vi "Checkers PvP With File Loading.vi"() -> ()   [LabVIEW 2016]
uses:
  <vilib>/Utility/miscctls.llb/LVPositionTypeDef.ctl
  Game Info Global Variable.vi
  Board Layout Global Variable.vi
panel:
  out "P2 Bottom Right Marker":picture
  out "P2 Bottom Left Marker":picture
  out "P2 Top Left Marker":picture
  out "P2 Top Right Marker":picture
  out "P1 Bottom Left Marker":picture
  out "P1 Bottom Right Marker":picture
  out "P1 Top Right Marker":picture
  out "P1 Top Left Marker":picture
  in  "Save and Quit":bool
  out "Player 2 Name":string="Player 2"
  out "Player 1 Name":string="Player 1"
  out "P2 King 12":picture
  out "P2 King 11":picture
  out "P2 King 10":picture
  out "P2 King 9":picture
  out "P2 King 8":picture
  out "P2 King 7":picture
  out "P2 King 6":picture
  out "P2 King 5":picture
  out "P2 King 4":picture
  out "P2 King 3":picture
  out "P2 King 2":picture
  out "P2 King":picture
  out "P1 King 12":picture
  out "P1 King 11":picture
  out "P1 King 10":picture
  out "P1 King 9":picture
  out "P1 King 8":picture
  out "P1 King 7":picture
  out "P1 King 6":picture
  out "P1 King 5":picture
  out "P1 King 4":picture
  out "P1 King 3":picture
  out "P1 King 2":picture
  out "P1 King":picture
  out "P2 Piece Icon":picture
  out "P1 Piece Icon":picture
  out "P2 Piece 12":picture
  out "P2 Piece 11":picture
  out "P2 Piece 10":picture
  out "P2 Piece 9":picture
  out "P2 Piece 8":picture
  out "P2 Piece 7":picture
  out "P2 Piece 6":picture
  out "P2 Piece 5":picture
  out "P2 Piece 4":picture
  out "P2 Piece 3":picture
  out "P2 Piece 2":picture
  out "P1 Piece 12":picture caption="P1 Piece"
  out "P1 Piece 11":picture caption="P1 Piece"
  out "P1 Piece 10":picture caption="P1 Piece"
  out "P1 Piece 9":picture caption="P1 Piece"
  out "P1 Piece 8":picture caption="P1 Piece"
  out "P1 Piece 7":picture caption="P1 Piece"
  out "P1 Piece 6":picture caption="P1 Piece"
  out "P1 Piece 5":picture caption="P1 Piece"
  out "P1 Piece 4":picture caption="P1 Piece"
  out "P1 Piece 3":picture caption="P1 Piece"
  out "P2 Piece":picture
  out "P1 Piece 2":picture caption="P1 Piece"
  out "Game String":string
  out "P2 Turn Light":bool
  out "P1 Turn Light":bool=TRUE
  out "P1 Piece":picture
  in  "Offer Draw":bool
  in  "Surrender":bool
  out "Player 2 Label":string="Player 1"
  out "Player 1 Label":string="Player 1"
  in  "Save":bool
  in  "Quit":bool
  # "Your Turn!"
  # "Your Turn!"
  # "678, \n308"
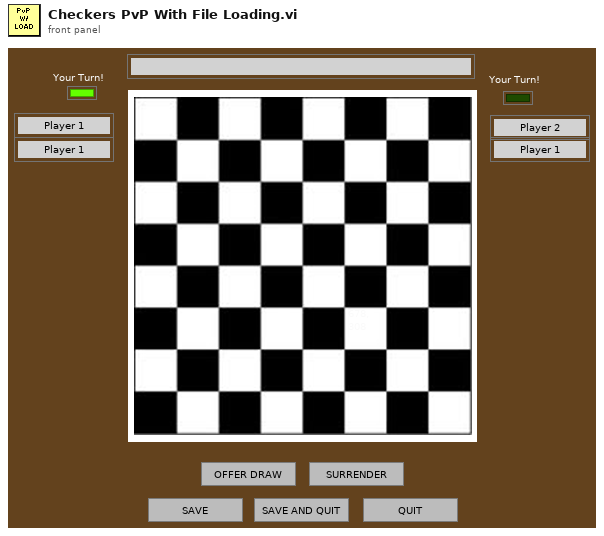
[diagram p1: front panel]
types:
  T1 = typedef "LVPositionTypeDef.ctl" = cluster{"Left":i32, "Top":i32}
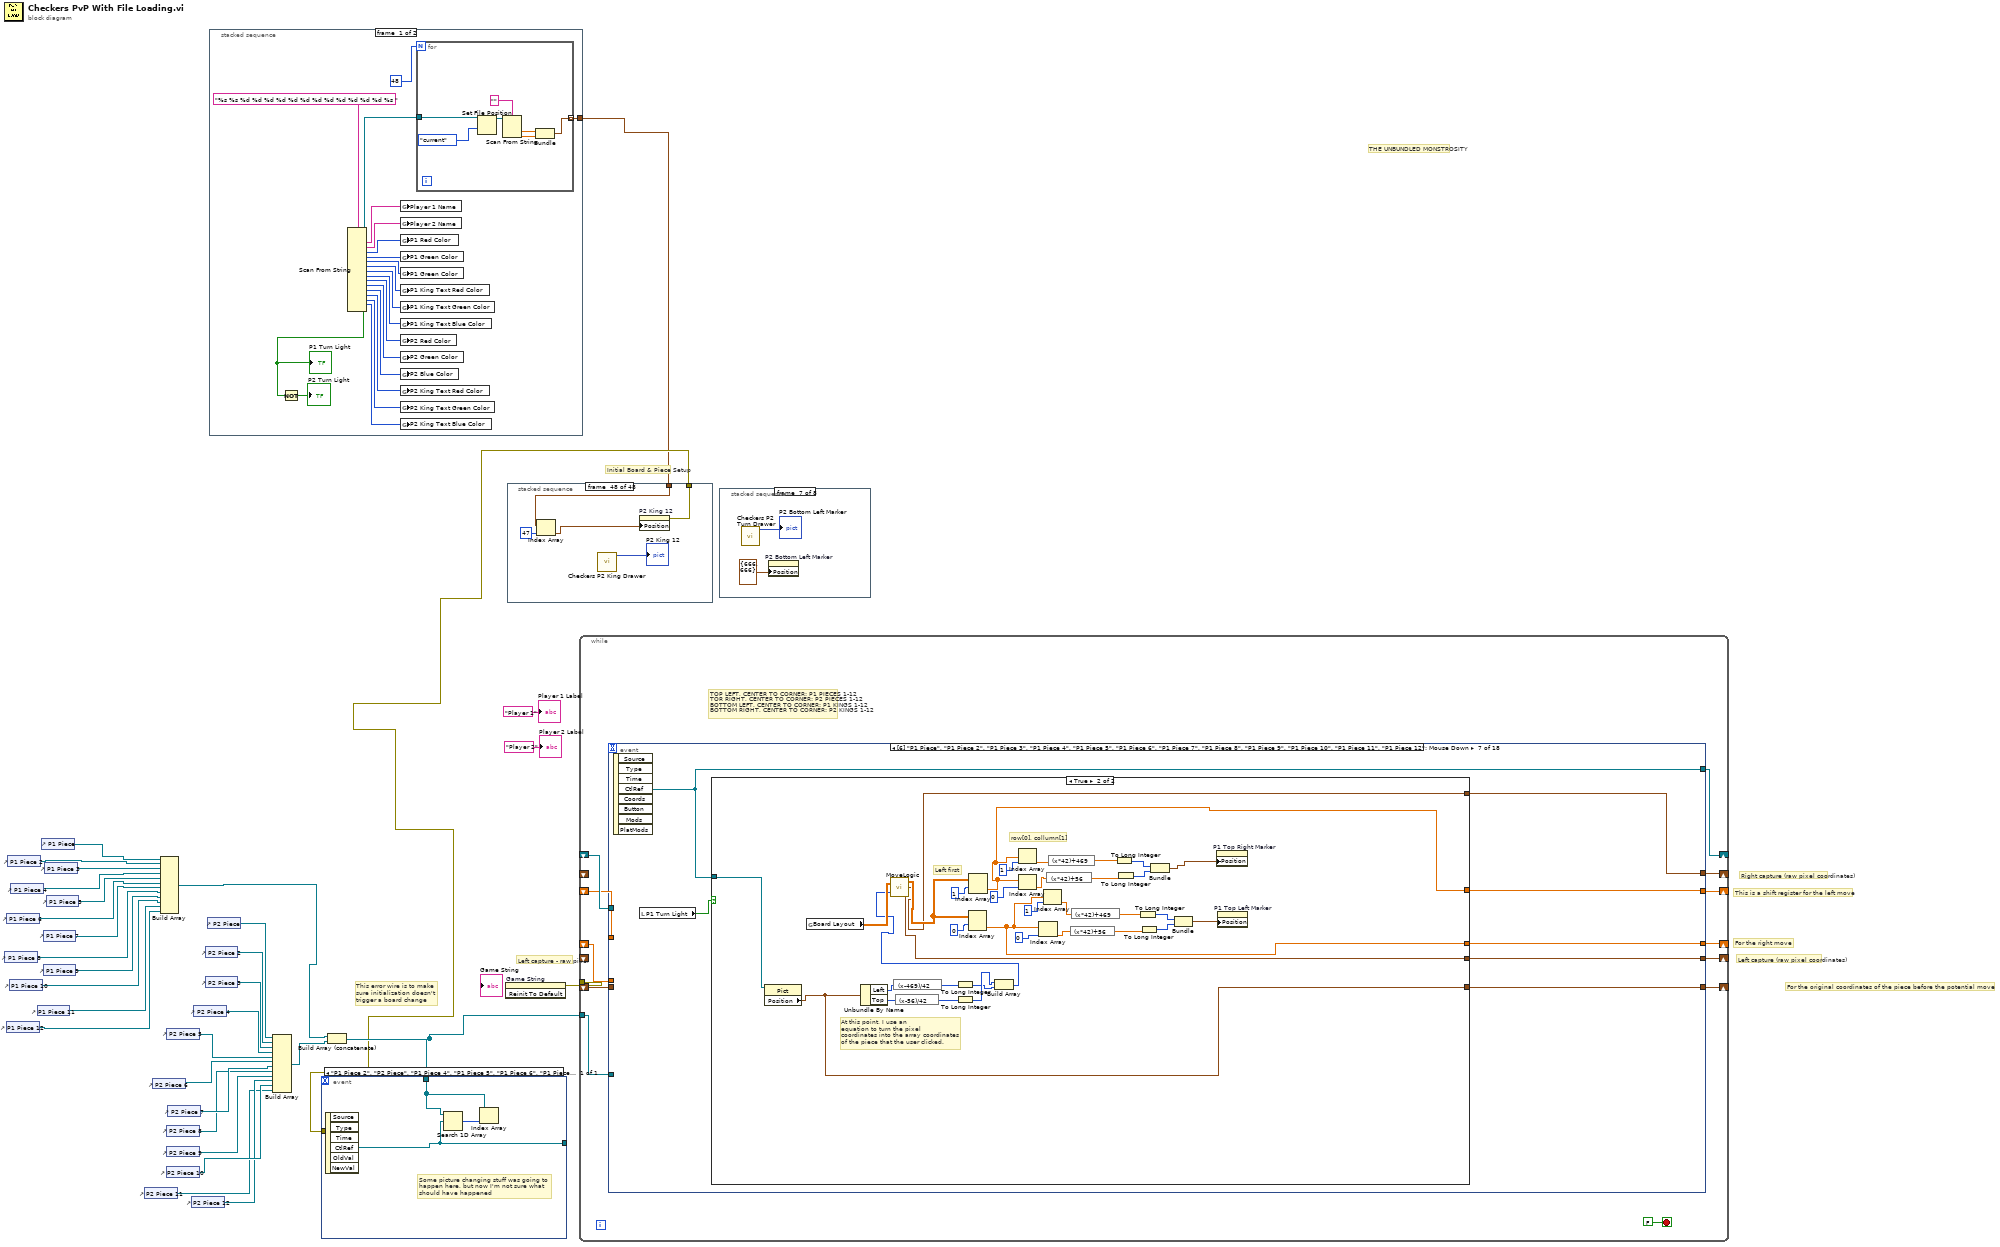
[diagram p0: block diagram]
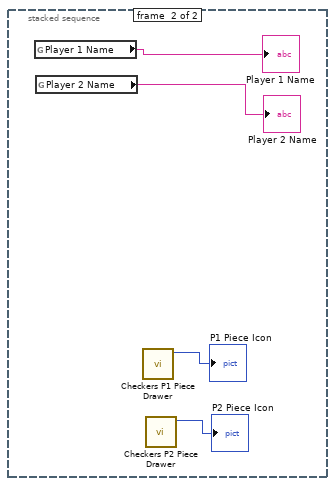
[diagram p2: hidden frame]
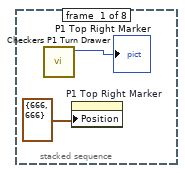
[diagram p3: hidden frame]
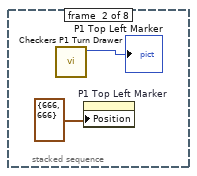
[diagram p4: hidden frame]
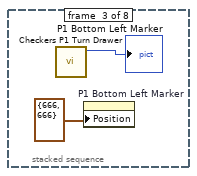
[diagram p5: hidden frame]
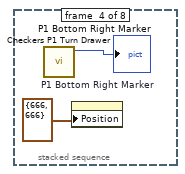
[diagram p6: hidden frame]
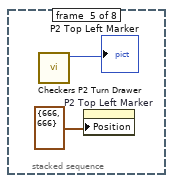
[diagram p7: hidden frame]
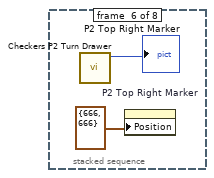
[diagram p8: hidden frame]
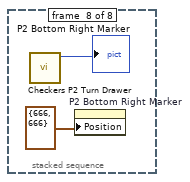
[diagram p9: hidden frame]
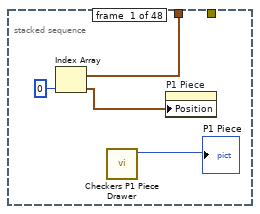
[diagram p10: hidden frame]
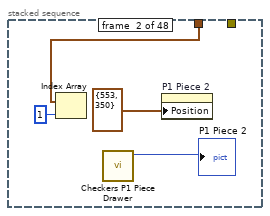
[diagram p11: hidden frame]
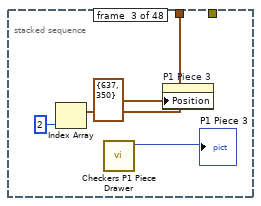
[diagram p12: hidden frame]
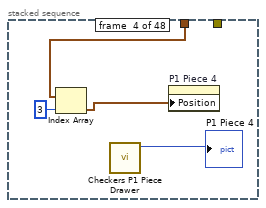
[diagram p13: hidden frame]
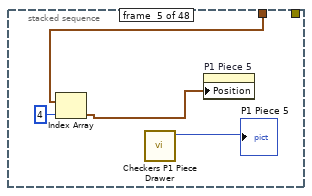
[diagram p14: hidden frame]
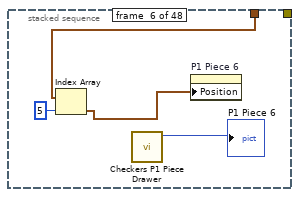
[diagram p15: hidden frame]
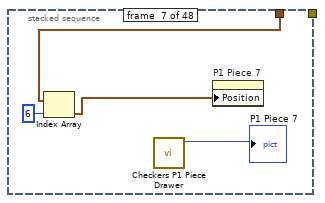
[diagram p16: hidden frame]
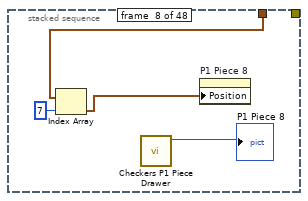
[diagram p17: hidden frame]
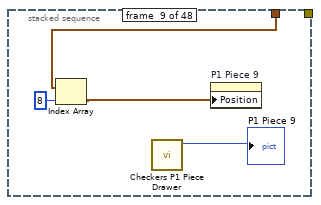
[diagram p18: hidden frame]
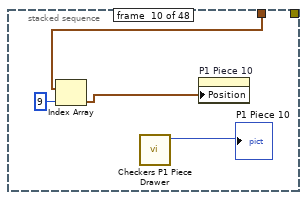
[diagram p19: hidden frame]
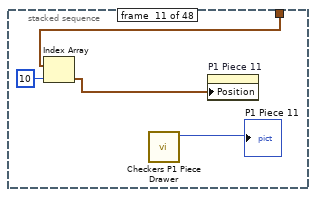
[diagram p20: hidden frame]
diagram:
  # "Left capture - raw pixel"
  # "Right capture (raw pixel coordinates)"
  # "Left capture (raw pixel coordinates)"
  # "For the original coordinates of the piece before the potential move"
  # "For the right move"
  # "This error wire is to make \nsure initialization doesn't \ntrigger a board change"
  # "This is a shift register for the left move"
  # "THE UNBUNDLED MONSTROSITY"
  # "Initial Board & Piece Setup"
  n1 = control-ref of="P1 Piece 8"() -> (w19:refnum<vi>)
  n2 = control-ref of="P1 Piece 6"() -> (w21:refnum<vi>)
  n3 = control-ref of="P1 Piece 12"() -> (w15:refnum<vi>)
  n4 = control-ref of="P1 Piece 2"() -> (w25:refnum<vi>)
  n5 = control-ref of="P1 Piece 10"() -> (w17:refnum<vi>)
  n6 = control-ref of="P1 Piece 4"() -> (w23:refnum<vi>)
  n7 = control-ref of="P1 Piece 11"() -> (w16:refnum<vi>)
  n8 = control-ref of="P1 Piece"() -> (w26:refnum<vi>)
  n9 = control-ref of="P1 Piece 7"() -> (w20:refnum<vi>)
  n10 = control-ref of="P1 Piece 9"() -> (w18:refnum<vi>)
  n11 = control-ref of="P1 Piece 3"() -> (w24:refnum<vi>)
  n12 = control-ref of="P1 Piece 5"() -> (w22:refnum<vi>)
  n13 = control-ref of="P2 Piece 11"() -> (w3:refnum<vi>)
  n14 = control-ref of="P2 Piece 6"() -> (w9:refnum<vi>)
  n15 = Build Array(w26, w25, w24, w23, w22, w21, w20, w19, w18, w17, w16, w15) -> (w2:refnum<vi>[])
  n16 = control-ref of="P2 Piece 5"() -> (w10:refnum<vi>)
  n17 = control-ref of="P2 Piece 8"() -> (w7:refnum<vi>)
  n18 = control-ref of="P2 Piece 9"() -> (w6:refnum<vi>)
  n19 = control-ref of="P2 Piece 10"() -> (w5:refnum<vi>)
  n20 = control-ref of="P2 Piece 7"() -> (w8:refnum<vi>)
  n21 = control-ref of="P2 Piece 12"() -> (w4:refnum<vi>)
  n22 = control-ref of="P2 Piece 4"() -> (w11:refnum<vi>)
  n23 = control-ref of="P2 Piece 2"() -> (w13:refnum<vi>)
  n24 = control-ref of="P2 Piece 3"() -> (w12:refnum<vi>)
  n25 = control-ref of="P2 Piece"() -> (w14:refnum<vi>)
  n26 = stacked-sequence {
    tunnel: [w35 _] -> w1
    frame #0 {
      n27 = Scan From String("%s %s %d %d %d %d %d %d %d %d %d %d %d %d %s " ("format string")) -> (w51:refnum<file>, output 1=w49:string, output 2=w48:string, output 3=w47:i32, output 4=w46:i32, output 5=w45:i32, output 6=w44:i32, output 7=w43:i32, output 8=w42:i32, output 9=w41:i32, output 10=w40:i32, output 11=w39:i32, output 12=w38:i32, output 13=w37:i32, output 14=w36:i32, output 15=w33:bool)  [unwired: 17 in, 1 out]
      "P1 Turn Light" <- w33
      n28 = Not(x=w33) -> (.not. x?=→"P2 Turn Light":bool)
      n29 = global write "Game Info Global Variable.vi" "Player 1 Name"(w49) -> ()
      n30 = global write "Game Info Global Variable.vi" "Player 2 Name"(w48) -> ()
      n31 = global write "Game Info Global Variable.vi" "P1 Red Color"(w47) -> ()
      n32 = global write "Game Info Global Variable.vi" "P1 Green Color"(w46) -> ()
      n33 = global write "Game Info Global Variable.vi" "P1 Green Color"(w45) -> ()
      n34 = global write "Game Info Global Variable.vi" "P1 King Text Red Color"(w44) -> ()
      n35 = global write "Game Info Global Variable.vi" "P1 King Text Green Color"(w43) -> ()
      n36 = global write "Game Info Global Variable.vi" "P1 King Text Blue Color"(w42) -> ()
      n37 = global write "Game Info Global Variable.vi" "P2 Red Color"(w41) -> ()
      n38 = global write "Game Info Global Variable.vi" "P2 Green Color"(w40) -> ()
      n39 = global write "Game Info Global Variable.vi" "P2 Blue Color"(w39) -> ()
      n40 = global write "Game Info Global Variable.vi" "P2 King Text Red Color"(w38) -> ()
      n41 = global write "Game Info Global Variable.vi" "P2 King Text Green Color"(w37) -> ()
      n42 = global write "Game Info Global Variable.vi" "P2 King Text Blue Color"(w36) -> ()
      n43 = for {
        N: 48 -> [_]
        tunnel: [w57] -> w35 mode=indexing
        tunnel: w51 -> [w55]
        n44 = Set File Position(refnum=w55, from (0:start)=enum16{"start", "end", "current"}."current") -> (refnum out=w54:refnum<file>)  [unwired: 2 in, 1 out]
        n45 = Scan From String("" ("format string"), w54) -> (output 1=w59:dbl, output 2=w58:dbl)  [unwired: 3 in, 2 out]
        n46 = Bundle(w59, w58) -> (w57:cluster{dbl, dbl})  [unwired: 1 in]
      }
    }
    frame #1 {
      n47 = global read "Game Info Global Variable.vi" "Player 1 Name"() -> (→"Player 1 Name":string)
      n48 = global read "Game Info Global Variable.vi" "Player 2 Name"() -> (→"Player 2 Name":string)
      n49 = call "Checkers P1 Piece Drawer.vi"() -> ("new picture"=→"P1 Piece Icon":picture)  [unwired: 11 in]
      n50 = call "Checkers P2 Piece Drawer.vi"() -> ("new picture"=→"P2 Piece Icon":picture)  [unwired: 11 in]
    }
  }
  n51 = Build Array(w14, w13, w12, w11, w10, w9, w8, w7, w6, w4, w5, w3) -> (w30:refnum<vi>[])
  n52 = Build Array (concatenate)(w2, w30) -> (w29:refnum<vi>[])
  n53 = invoke on="Game String" class="Str" method="Reinit To Default"() -> (error out=w31:errorcluster)  [unwired: 3 in, 2 out]
  n54 = stacked-sequence {
    tunnel: [_ _ _ _ _ _ _ _ _ _ _ _ _ _ _ _ _ _ _ _ _ _ _ _ _ _ _ _ _ _ _ _ _ _ _ _ _ _ _ _ _ _ _ _ _ _ _ w255] -> w27
    tunnel: w1 -> [w66 w68 w72 w77 w81 w85 w88 w93 w97 w101 w104 w109 w113 w117 w121 w125 w129 w133 w137 w141 w145 w149 w153 w156 w161 w165 w169 w173 w176 w181 w185 w189 w193 w197 w201 w205 w209 w213 w217 w221 w225 w229 w233 w237 w241 w245 w249 w253]
    frame #0 {
      n55 = Index Array(array=w66, index=0) -> (element=w64:cluster{dbl, dbl})
      n56 = call "Checkers P1 Piece Drawer.vi"() -> ("new picture"=→"P1 Piece":picture)  [unwired: 11 in]
      n57 = property on="P1 Piece" class="Pict"("Position"=w64) -> ()  [unwired: 2 in, 2 out]
    }
    frame #1 {
      n58 = Index Array(array=w68, index=1) -> ()  [unwired: 1 out]
      n59 = call "Checkers P1 Piece Drawer.vi"() -> ("new picture"=→"P1 Piece 2":picture)  [unwired: 11 in]
      n60 = property on="P1 Piece 2" class="Pict"("Position"=T1 {"Left"=553, "Top"=350}) -> ()  [unwired: 2 in, 2 out]
    }
    frame #2 {
      n61 = Index Array(array=w72, index=2) -> ()  [unwired: 1 out]
      n62 = call "Checkers P1 Piece Drawer.vi"() -> ("new picture"=→"P1 Piece 3":picture)  [unwired: 11 in]
      n63 = property on="P1 Piece 3" class="Pict"("Position"=T1 {"Left"=637, "Top"=350}) -> ()  [unwired: 2 in, 2 out]
    }
    frame #3 {
      n64 = Index Array(array=w77, index=3) -> (element=w76:cluster{dbl, dbl})
      n65 = call "Checkers P1 Piece Drawer.vi"() -> ("new picture"=→"P1 Piece 4":picture)  [unwired: 11 in]
      n66 = property on="P1 Piece 4" class="Pict"("Position"=w76) -> ()  [unwired: 2 in, 2 out]
    }
    frame #4 {
      n67 = Index Array(array=w81, index=4) -> (element=w80:cluster{dbl, dbl})
      n68 = call "Checkers P1 Piece Drawer.vi"() -> ("new picture"=→"P1 Piece 5":picture)  [unwired: 11 in]
      n69 = property on="P1 Piece 5" class="Pict"("Position"=w80) -> ()  [unwired: 2 in, 2 out]
    }
    frame #5 {
      n70 = Index Array(array=w85, index=5) -> (element=w84:cluster{dbl, dbl})
      n71 = call "Checkers P1 Piece Drawer.vi"() -> ("new picture"=→"P1 Piece 6":picture)  [unwired: 11 in]
      n72 = property on="P1 Piece 6" class="Pict"("Position"=w84) -> ()  [unwired: 2 in, 2 out]
    }
    frame #6 {
      n73 = Index Array(array=w88, index=6) -> (element=w89:cluster{dbl, dbl})
      n74 = call "Checkers P1 Piece Drawer.vi"() -> ("new picture"=→"P1 Piece 7":picture)  [unwired: 11 in]
      n75 = property on="P1 Piece 7" class="Pict"("Position"=w89) -> ()  [unwired: 2 in, 2 out]
    }
    frame #7 {
      n76 = Index Array(array=w93, index=7) -> (element=w92:cluster{dbl, dbl})
      n77 = call "Checkers P1 Piece Drawer.vi"() -> ("new picture"=→"P1 Piece 8":picture)  [unwired: 11 in]
      n78 = property on="P1 Piece 8" class="Pict"("Position"=w92) -> ()  [unwired: 2 in, 2 out]
    }
    frame #8 {
      n79 = Index Array(array=w97, index=8) -> (element=w96:cluster{dbl, dbl})
      n80 = call "Checkers P1 Piece Drawer.vi"() -> ("new picture"=→"P1 Piece 9":picture)  [unwired: 11 in]
      n81 = property on="P1 Piece 9" class="Pict"("Position"=w96) -> ()  [unwired: 2 in, 2 out]
    }
    frame #9 {
      n82 = Index Array(array=w101, index=9) -> (element=w100:cluster{dbl, dbl})
      n83 = call "Checkers P1 Piece Drawer.vi"() -> ("new picture"=→"P1 Piece 10":picture)  [unwired: 11 in]
      n84 = property on="P1 Piece 10" class="Pict"("Position"=w100) -> ()  [unwired: 2 in, 2 out]
    }
    frame #10 {
      n85 = Index Array(array=w104, index=10) -> (element=w105:cluster{dbl, dbl})
      n86 = call "Checkers P1 Piece Drawer.vi"() -> ("new picture"=→"P1 Piece 11":picture)  [unwired: 11 in]
      n87 = property on="P1 Piece 11" class="Pict"("Position"=w105) -> ()  [unwired: 2 in, 2 out]
    }
    frame #11 {
      n88 = Index Array(array=w109, index=11) -> (element=w108:cluster{dbl, dbl})
      n89 = call "Checkers P1 Piece Drawer.vi"() -> ("new picture"=→"P1 Piece 12":picture)  [unwired: 11 in]
      n90 = property on="P1 Piece 12" class="Pict"("Position"=w108) -> ()  [unwired: 2 in, 2 out]
    }
    frame #12 {
      n91 = Index Array(array=w113, index=12) -> (element=w112:cluster{dbl, dbl})
      n92 = call "Checkers P2 Piece Drawer.vi"() -> ("new picture"=→"P2 Piece":picture)  [unwired: 11 in]
      n93 = property on="P2 Piece" class="Pict"("Position"=w112) -> ()  [unwired: 2 in, 2 out]
    }
    frame #13 {
      n94 = Index Array(array=w117, index=13) -> (element=w116:cluster{dbl, dbl})
      n95 = call "Checkers P2 Piece Drawer.vi"() -> ("new picture"=→"P2 Piece 2":picture)  [unwired: 11 in]
      n96 = property on="P2 Piece 2" class="Pict"("Position"=w116) -> ()  [unwired: 2 in, 2 out]
    }
    frame #14 {
      n97 = Index Array(array=w121, index=14) -> (element=w120:cluster{dbl, dbl})
      n98 = call "Checkers P2 Piece Drawer.vi"() -> ("new picture"=→"P2 Piece 3":picture)  [unwired: 11 in]
      n99 = property on="P2 Piece 3" class="Pict"("Position"=w120) -> ()  [unwired: 2 in, 2 out]
    }
    frame #15 {
      n100 = Index Array(array=w125, index=15) -> (element=w124:cluster{dbl, dbl})
      n101 = call "Checkers P2 Piece Drawer.vi"() -> ("new picture"=→"P2 Piece 4":picture)  [unwired: 11 in]
      n102 = property on="P2 Piece 4" class="Pict"("Position"=w124) -> ()  [unwired: 2 in, 2 out]
    }
    frame #16 {
      n103 = Index Array(array=w129, index=16) -> (element=w128:cluster{dbl, dbl})
      n104 = call "Checkers P2 Piece Drawer.vi"() -> ("new picture"=→"P2 Piece 5":picture)  [unwired: 11 in]
      n105 = property on="P2 Piece 5" class="Pict"("Position"=w128) -> ()  [unwired: 2 in, 2 out]
    }
    frame #17 {
      n106 = Index Array(array=w133, index=17) -> (element=w132:cluster{dbl, dbl})
      n107 = call "Checkers P2 Piece Drawer.vi"() -> ("new picture"=→"P2 Piece 6":picture)  [unwired: 11 in]
      n108 = property on="P2 Piece 6" class="Pict"("Position"=w132) -> ()  [unwired: 2 in, 2 out]
    }
    frame #18 {
      n109 = Index Array(array=w137, index=18) -> (element=w136:cluster{dbl, dbl})
      n110 = call "Checkers P2 Piece Drawer.vi"() -> ("new picture"=→"P2 Piece 7":picture)  [unwired: 11 in]
      n111 = property on="P2 Piece 7" class="Pict"("Position"=w136) -> ()  [unwired: 2 in, 2 out]
    }
    frame #19 {
      n112 = Index Array(array=w141, index=19) -> (element=w140:cluster{dbl, dbl})
      n113 = call "Checkers P2 Piece Drawer.vi"() -> ("new picture"=→"P2 Piece 8":picture)  [unwired: 11 in]
      n114 = property on="P2 Piece 8" class="Pict"("Position"=w140) -> ()  [unwired: 2 in, 2 out]
    }
    frame #20 {
      n115 = Index Array(array=w145, index=20) -> (element=w144:cluster{dbl, dbl})
      n116 = call "Checkers P2 Piece Drawer.vi"() -> ("new picture"=→"P2 Piece 9":picture)  [unwired: 11 in]
      n117 = property on="P2 Piece 9" class="Pict"("Position"=w144) -> ()  [unwired: 2 in, 2 out]
    }
    frame #21 {
      n118 = Index Array(array=w149, index=21) -> (element=w148:cluster{dbl, dbl})
      n119 = call "Checkers P2 Piece Drawer.vi"() -> ("new picture"=→"P2 Piece 10":picture)  [unwired: 11 in]
      n120 = property on="P2 Piece 10" class="Pict"("Position"=w148) -> ()  [unwired: 2 in, 2 out]
    }
    frame #22 {
      n121 = Index Array(array=w153, index=22) -> (element=w152:cluster{dbl, dbl})
      n122 = call "Checkers P2 Piece Drawer.vi"() -> ("new picture"=→"P2 Piece 11":picture)  [unwired: 11 in]
      n123 = property on="P2 Piece 11" class="Pict"("Position"=w152) -> ()  [unwired: 2 in, 2 out]
    }
    frame #23 {
      n124 = Index Array(array=w156, index=23) -> (element=w157:cluster{dbl, dbl})
      n125 = call "Checkers P2 Piece Drawer.vi"() -> ("new picture"=→"P2 Piece 12":picture)  [unwired: 11 in]
      n126 = property on="P2 Piece 12" class="Pict"("Position"=w157) -> ()  [unwired: 2 in, 2 out]
    }
    frame #24 {
      n127 = Index Array(array=w161, index=24) -> (element=w160:cluster{dbl, dbl})
      n128 = call "Checkers P1 King Drawer.vi"() -> ("new picture"=→"P1 King":picture)  [unwired: 11 in]
      n129 = property on="P1 King" class="Pict"("Position"=w160) -> ()  [unwired: 2 in, 2 out]
    }
    frame #25 {
      n130 = Index Array(array=w165, index=25) -> (element=w164:cluster{dbl, dbl})
      n131 = call "Checkers P1 King Drawer.vi"() -> ("new picture"=→"P1 King 2":picture)  [unwired: 11 in]
      n132 = property on="P1 King 2" class="Pict"("Position"=w164) -> ()  [unwired: 2 in, 2 out]
    }
    frame #26 {
      n133 = Index Array(array=w169, index=26) -> (element=w168:cluster{dbl, dbl})
      n134 = call "Checkers P1 King Drawer.vi"() -> ("new picture"=→"P1 King 3":picture)  [unwired: 11 in]
      n135 = property on="P1 King 3" class="Pict"("Position"=w168) -> ()  [unwired: 2 in, 2 out]
    }
    frame #27 {
      n136 = Index Array(array=w173, index=27) -> (element=w172:cluster{dbl, dbl})
      n137 = call "Checkers P1 King Drawer.vi"() -> ("new picture"=→"P1 King 4":picture)  [unwired: 11 in]
      n138 = property on="P1 King 4" class="Pict"("Position"=w172) -> ()  [unwired: 2 in, 2 out]
    }
    frame #28 {
      n139 = Index Array(array=w176, index=28) -> (element=w177:cluster{dbl, dbl})
      n140 = call "Checkers P1 King Drawer.vi"() -> ("new picture"=→"P1 King 5":picture)  [unwired: 11 in]
      n141 = property on="P1 King 5" class="Pict"("Position"=w177) -> ()  [unwired: 2 in, 2 out]
    }
    frame #29 {
      n142 = Index Array(array=w181, index=29) -> (element=w180:cluster{dbl, dbl})
      n143 = call "Checkers P1 King Drawer.vi"() -> ("new picture"=→"P1 King 6":picture)  [unwired: 11 in]
      n144 = property on="P1 King 6" class="Pict"("Position"=w180) -> ()  [unwired: 2 in, 2 out]
    }
    frame #30 {
      n145 = Index Array(array=w185, index=30) -> (element=w184:cluster{dbl, dbl})
      n146 = call "Checkers P1 King Drawer.vi"() -> ("new picture"=→"P1 King 7":picture)  [unwired: 11 in]
      n147 = property on="P1 King 7" class="Pict"("Position"=w184) -> ()  [unwired: 2 in, 2 out]
    }
    frame #31 {
      n148 = Index Array(array=w189, index=31) -> (element=w188:cluster{dbl, dbl})
      n149 = call "Checkers P1 King Drawer.vi"() -> ("new picture"=→"P1 King 8":picture)  [unwired: 11 in]
      n150 = property on="P1 King 8" class="Pict"("Position"=w188) -> ()  [unwired: 2 in, 2 out]
    }
    frame #32 {
      n151 = Index Array(array=w193, index=32) -> (element=w192:cluster{dbl, dbl})
      n152 = call "Checkers P1 King Drawer.vi"() -> ("new picture"=→"P1 King 9":picture)  [unwired: 11 in]
      n153 = property on="P1 King 9" class="Pict"("Position"=w192) -> ()  [unwired: 2 in, 2 out]
    }
    frame #33 {
      n154 = Index Array(array=w197, index=33) -> (element=w196:cluster{dbl, dbl})
      n155 = call "Checkers P1 King Drawer.vi"() -> ("new picture"=→"P1 King 10":picture)  [unwired: 11 in]
      n156 = property on="P1 King 10" class="Pict"("Position"=w196) -> ()  [unwired: 2 in, 2 out]
    }
    frame #34 {
      n157 = Index Array(array=w201, index=34) -> (element=w200:cluster{dbl, dbl})
      n158 = call "Checkers P1 King Drawer.vi"() -> ("new picture"=→"P1 King 11":picture)  [unwired: 11 in]
      n159 = property on="P1 King 11" class="Pict"("Position"=w200) -> ()  [unwired: 2 in, 2 out]
    }
    frame #35 {
      n160 = Index Array(array=w205, index=35) -> (element=w204:cluster{dbl, dbl})
      n161 = call "Checkers P1 King Drawer.vi"() -> ("new picture"=→"P1 King 12":picture)  [unwired: 11 in]
      n162 = property on="P1 King 12" class="Pict"("Position"=w204) -> ()  [unwired: 2 in, 2 out]
    }
    frame #36 {
      n163 = Index Array(array=w209, index=36) -> (element=w208:cluster{dbl, dbl})
      n164 = call "Checkers P2 King Drawer.vi"() -> ("new picture"=→"P2 King":picture)  [unwired: 11 in]
      n165 = property on="P2 King" class="Pict"("Position"=w208) -> ()  [unwired: 2 in, 2 out]
    }
    frame #37 {
      n166 = Index Array(array=w213, index=37) -> (element=w212:cluster{dbl, dbl})
      n167 = call "Checkers P2 King Drawer.vi"() -> ("new picture"=→"P2 King 2":picture)  [unwired: 11 in]
      n168 = property on="P2 King 2" class="Pict"("Position"=w212) -> ()  [unwired: 2 in, 2 out]
    }
    frame #38 {
      n169 = Index Array(array=w217, index=38) -> (element=w216:cluster{dbl, dbl})
      n170 = call "Checkers P2 King Drawer.vi"() -> ("new picture"=→"P2 King 3":picture)  [unwired: 11 in]
      n171 = property on="P2 King 3" class="Pict"("Position"=w216) -> ()  [unwired: 2 in, 2 out]
    }
    frame #39 {
      n172 = Index Array(array=w221, index=39) -> (element=w220:cluster{dbl, dbl})
      n173 = call "Checkers P2 King Drawer.vi"() -> ("new picture"=→"P2 King 4":picture)  [unwired: 11 in]
      n174 = property on="P2 King 4" class="Pict"("Position"=w220) -> ()  [unwired: 2 in, 2 out]
    }
    frame #40 {
      n175 = Index Array(array=w225, index=40) -> (element=w224:cluster{dbl, dbl})
      n176 = call "Checkers P2 King Drawer.vi"() -> ("new picture"=→"P2 King 5":picture)  [unwired: 11 in]
      n177 = property on="P2 King 5" class="Pict"("Position"=w224) -> ()  [unwired: 2 in, 2 out]
    }
    frame #41 {
      n178 = Index Array(array=w229, index=41) -> (element=w228:cluster{dbl, dbl})
      n179 = call "Checkers P2 King Drawer.vi"() -> ("new picture"=→"P2 King 6":picture)  [unwired: 11 in]
      n180 = property on="P2 King 6" class="Pict"("Position"=w228) -> ()  [unwired: 2 in, 2 out]
    }
    frame #42 {
      n181 = Index Array(array=w233, index=42) -> (element=w232:cluster{dbl, dbl})
      n182 = call "Checkers P2 King Drawer.vi"() -> ("new picture"=→"P2 King 7":picture)  [unwired: 11 in]
      n183 = property on="P2 King 7" class="Pict"("Position"=w232) -> ()  [unwired: 2 in, 2 out]
    }
    frame #43 {
      n184 = Index Array(array=w237, index=43) -> (element=w236:cluster{dbl, dbl})
      n185 = call "Checkers P2 King Drawer.vi"() -> ("new picture"=→"P2 King 8":picture)  [unwired: 11 in]
      n186 = property on="P2 King 8" class="Pict"("Position"=w236) -> ()  [unwired: 2 in, 2 out]
    }
    frame #44 {
      n187 = Index Array(array=w241, index=44) -> (element=w240:cluster{dbl, dbl})
      n188 = call "Checkers P2 King Drawer.vi"() -> ("new picture"=→"P2 King 9":picture)  [unwired: 11 in]
      n189 = property on="P2 King 9" class="Pict"("Position"=w240) -> ()  [unwired: 2 in, 2 out]
    }
    frame #45 {
      n190 = Index Array(array=w245, index=45) -> (element=w244:cluster{dbl, dbl})
      n191 = call "Checkers P2 King Drawer.vi"() -> ("new picture"=→"P2 King 10":picture)  [unwired: 11 in]
      n192 = property on="P2 King 10" class="Pict"("Position"=w244) -> ()  [unwired: 2 in, 2 out]
    }
    frame #46 {
      n193 = Index Array(array=w249, index=46) -> (element=w248:cluster{dbl, dbl})
      n194 = call "Checkers P2 King Drawer.vi"() -> ("new picture"=→"P2 King 11":picture)  [unwired: 11 in]
      n195 = property on="P2 King 11" class="Pict"("Position"=w248) -> ()  [unwired: 2 in, 2 out]
    }
    frame #47 {
      n196 = Index Array(array=w253, index=47) -> (element=w252:cluster{dbl, dbl})
      n197 = call "Checkers P2 King Drawer.vi"() -> ("new picture"=→"P2 King 12":picture)  [unwired: 11 in]
      n198 = property on="P2 King 12" class="Pict"("Position"=w252) -> (error out=w255:errorcluster)  [unwired: 2 in, 1 out]
    }
  }
  n199 = event shown="[0] \"P1 Piece 2\", \"P2 Piece\", \"P1 Piece 4\", \"P1 Piece 5\", \"P1 Piece 6\", \"P1 Piece 7\", \"P1 Piece 8\", \"P1 Piece 9\", \"P1 Piece 10\", \"P1 Piece 11\", \"P1 Piece 12\", \"P2 Piece 2\", \"P2 Piece 3\", \"P2 Piece 4\", \"P2 Piece 6\", \"P2 Piece 7\", \"P2 Piece 8\", \"P2 Piece 9\", \"P2 Piece 10\", \"P2 Piece 11\", \"P2 Piece 12\": Value Change" {
    selector: _ -> [_]
    dyn-events: _ -> [_]
    timeout: _ -> [_]
    tunnel: [w259] -> _
    tunnel: w29 -> [w258]
    tunnel: w27 -> [_]
    event "P1 Piece 2", "P2 Piece", "P1 Piece 4", "P1 Piece 5", "P1 Piece 6", "P1 Piece 7", "P1 Piece 8", "P1 Piece 9", "P1 Piece 10", "P1 Piece 11", "P1 Piece 12", "P2 Piece 2", "P2 Piece 3", "P2 Piece 4", "P2 Piece 6", "P2 Piece 7", "P2 Piece 8", "P2 Piece 9", "P2 Piece 10", "P2 Piece 11", "P2 Piece 12": Value Change {
      # "Some picture changing stuff was going to \nhappen here, but now I'm not sure what \nshould have happened"
      n200 = event-data() -> ("CtlRef"=w259:refnum<vi>)  [unwired: 1 in, 5 out]
      n201 = Search 1D Array(1D array=w258, element=w259) -> (index of element=w257:i32)  [unwired: 1 in]
      n202 = Index Array(array=w258, index=w257) -> ()  [unwired: 1 out]
    }
  }
  n203 = while {
    tunnel: w31 -> [_]
    tunnel: w29 -> [w261]
    shift-right: [w271] -> _
    shift-left: _ -> [w270]
    shift-right: [w269] -> _
    shift-left: _ -> [w264]
    shift-right: [w268] -> _
    shift-left: _ -> [w267]
    shift-right: [w266] -> _
    shift-left: _ -> [w265]
    shift-right: [w263] -> _
    shift-left: _ -> [_]
    shift-right: [w262] -> _
    shift-left: _ -> [_]
    stop <- FALSE stop-if-true
    # "TOP LEFT, CENTER TO CORNER: P1 PIECES 1-12\nTOR RIGHT, CENTER TO CORNER: P2 PIECES 1-12\nBOTTOM LEFT, CENTER TO CORNER: P1 KINGS 1-12\nBOTTOM RIGHT, CENTER TO CORNER: P2 KINGS 1-12"
    n204 = event shown="[6] \"P1 Piece\", \"P1 Piece 2\", \"P1 Piece 3\", \"P1 Piece 4\", \"P1 Piece 5\", \"P1 Piece 6\", \"P1 Piece 7\", \"P1 Piece 8\", \"P1 Piece 9\", \"P1 Piece 10\", \"P1 Piece 11\", \"P1 Piece 12\": Mouse Down" {
      selector: _ -> [_ _ _ _ _ _ _ _ _ _ _ _ _ _ _ _ _ _]
      dyn-events: _ -> [_ _ _ _ _ _ _ _ _ _ _ _ _ _ _ _ _ _]
      timeout: _ -> [_ _ _ _ _ _ _ _ _ _ _ _ _ _ _ _ _ _]
      tunnel: [_ _ _ _ _ _ w647 w684 w724 w760 _ _ _ _ _ _ _ _] -> w271
      tunnel: w270 -> [_ _ _ _ _ _ _ _ _ _ w890 w901 w912 w923 w934 w949 w984 w1075]
      tunnel: [_ _ _ _ _ _ w646 _ w722 _ _ _ _ _ _ _ _ _] -> w269
      tunnel: [_ _ _ _ _ _ w645 _ w723 _ _ _ _ _ _ _ _ _] -> w268
      tunnel: w267 -> [_ _ _ _ _ _ _ _ _ _ w884 _ _ _ _ _ _ _]
      tunnel: [_ _ _ _ _ _ w644 _ w720 _ _ _ _ _ _ _ _ _] -> w266
      tunnel: w265 -> [_ _ _ _ _ _ _ _ _ _ w883 _ _ _ _ w936 _ _]
      tunnel: w264 -> [_ _ _ _ _ _ _ _ _ _ _ _ _ _ _ w935 _ _]
      tunnel: [_ _ _ _ _ _ w643 _ w721 _ _ _ _ _ _ _ _ _] -> w263
      tunnel: [_ _ _ _ _ _ w642 _ _ _ _ _ _ _ _ _ _ _] -> w262
      tunnel: w261 -> [_ _ _ _ _ _ _ _ _ _ w796 _ _ _ _ _ _ _]
      event Timeout {
        n205 = event-data() -> ()  [unwired: 1 in, 3 out]
      }
      event "Offer Draw": Value Change {
        n206 = event-data() -> ()  [unwired: 1 in, 6 out]
        n207 = local read "P1 Turn Light"() -> (w272:bool)
        n208 = case shown="False" w272 {
          frame False {
            n209 = local read "Player 2 Name"() -> (w276:string)
            n210 = Format Into String(format string="%s offers a stalemate. Do you accept?", w276) -> (resulting string=w274:string)  [unwired: 2 in, 1 out]
            n211 = Two Button Dialog(message=w274, 1:"Decline" ("F button name (\"Cancel\")"), 2:"Accept" ("T button name (\"OK\")")) -> (T button?=w273:bool)
            n212 = case shown="True" w273 {
              frame False {
                # "Stalemate offer rejected. Do nothing."
              }
              frame True {
                w279 = "GAME OVER. It's a draw." ("format string")
                n213 = local write "Game String"(w279) -> ()
                n214 = Two Button Dialog(message=w279, 1:"Main Menu" ("F button name (\"Cancel\")"), 2:"New Game" ("T button name (\"OK\")")) -> (T button?=w282:bool)
                n215 = case shown="False" w282 {
                  frame False {
                    n216 = vi-ref "Checkers Main Menu.vi"() -> (w289:refnum<vi>)
                    n217 = invoke class="VI" method="Run VI"(reference=w289, "Wait until done"=FALSE ("Wait Until Done")) -> (reference out=w288:refnum<vi>, error out=w287:errorcluster)  [unwired: 3 in, 3 out]
                    n218 = invoke class="VI" method="FP.Open"(reference=w288, error in=w287, "Activate"=TRUE ("Activate?")) -> (error out=w286:errorcluster)  [unwired: 2 in, 4 out]
                    n219 = vi-ref "Checkers PvP With File Loading.vi"() -> (w285:refnum<vi>)
                    n220 = invoke class="VI" method="Abort VI"(reference=w285, error in=w286) -> ()  [unwired: 1 in, 3 out]
                  }
                  frame True {
                    n221 = vi-ref "Checkers New Game.vi"() -> (w296:refnum<vi>)
                    n222 = invoke class="VI" method="Run VI"(reference=w296, "Wait until done"=FALSE ("Wait Until Done")) -> (reference out=w295:refnum<vi>, error out=w294:errorcluster)  [unwired: 3 in, 3 out]
                    n223 = invoke class="VI" method="FP.Open"(reference=w295, error in=w294, "Activate"=TRUE ("Activate?")) -> (error out=w293:errorcluster)  [unwired: 2 in, 4 out]
                    n224 = vi-ref "Checkers PvP With File Loading.vi"() -> (w292:refnum<vi>)
                    n225 = invoke class="VI" method="Abort VI"(reference=w292, error in=w293) -> ()  [unwired: 1 in, 3 out]
                  }
                }
              }
            }
          }
          frame True {
            n226 = local read "Player 1 Name"() -> (w300:string)
            n227 = Format Into String(format string="%s offers a stalemate. Do you accept?", w300) -> (resulting string=w298:string)  [unwired: 2 in, 1 out]
            n228 = Two Button Dialog(message=w298, 1:"Decline" ("F button name (\"Cancel\")"), 2:"Accept" ("T button name (\"OK\")")) -> (T button?=w297:bool)
            n229 = case shown="True" w297 {
              frame False {
                # "Stalemate offer was rejected. Do nothing."
              }
              frame True {
                w303 = "GAME OVER. Stalemate." ("format string")
                n230 = local write "Game String"(w303) -> ()
                n231 = Two Button Dialog(message=w303, 1:"Main Menu" ("F button name (\"Cancel\")"), 2:"New Game" ("T button name (\"OK\")")) -> (T button?=w306:bool)
                n232 = case shown="False" w306 {
                  frame False {
                    n233 = vi-ref "Checkers Main Menu.vi"() -> (w313:refnum<vi>)
                    n234 = invoke class="VI" method="Run VI"(reference=w313, "Wait until done"=FALSE ("Wait Until Done")) -> (reference out=w312:refnum<vi>, error out=w311:errorcluster)  [unwired: 3 in, 3 out]
                    n235 = invoke class="VI" method="FP.Open"(reference=w312, error in=w311, "Activate"=TRUE ("Activate?")) -> (error out=w310:errorcluster)  [unwired: 2 in, 4 out]
                    n236 = vi-ref "Checkers PvP With File Loading.vi"() -> (w309:refnum<vi>)
                    n237 = invoke class="VI" method="Abort VI"(reference=w309, error in=w310) -> ()  [unwired: 1 in, 3 out]
                  }
                  frame True {
                    n238 = vi-ref "Checkers New Game.vi"() -> (w320:refnum<vi>)
                    n239 = invoke class="VI" method="Run VI"(reference=w320, "Wait until done"=FALSE ("Wait Until Done")) -> (reference out=w319:refnum<vi>, error out=w318:errorcluster)  [unwired: 3 in, 3 out]
                    n240 = invoke class="VI" method="FP.Open"(reference=w319, error in=w318, "Activate"=TRUE ("Activate?")) -> (error out=w317:errorcluster)  [unwired: 2 in, 4 out]
                    n241 = vi-ref "Checkers PvP With File Loading.vi"() -> (w316:refnum<vi>)
                    n242 = invoke class="VI" method="Abort VI"(reference=w316, error in=w317) -> ()  [unwired: 1 in, 3 out]
                  }
                }
              }
            }
          }
        }
      }
      event "Surrender": Value Change {
        n243 = event-data() -> ()  [unwired: 1 in, 6 out]
        n244 = Two Button Dialog(message="Are you sure you want to surrender?", 1:"No" ("F button name (\"Cancel\")"), 2:"Yes" ("T button name (\"OK\")")) -> (T button?=w321:bool)
        n245 = case shown="True" w321 {
          frame False {
            # "Player changed mind, didn't surrender. Do nothing."
          }
          frame True {
            n246 = local read "P1 Turn Light"() -> (w325:bool)
            n247 = case shown="True" w325 {
              frame False {
                n248 = local read "Player 1 Name"() -> (w326:string)
                n249 = Format Into String(format string="GAME OVER. %s WINS!", w326) -> (resulting string=w330:string)  [unwired: 2 in, 1 out]
                n250 = local write "Game String"(w330) -> ()
                n251 = Two Button Dialog(message=w330, 1:"Main Menu" ("F button name (\"Cancel\")"), 2:"New Game" ("T button name (\"OK\")")) -> (T button?=w327:bool)
                n252 = case shown="True" w327 {
                  frame False {
                    n253 = vi-ref "Checkers Main Menu.vi"() -> (w338:refnum<vi>)
                    n254 = invoke class="VI" method="Run VI"(reference=w338, "Wait until done"=FALSE ("Wait Until Done")) -> (reference out=w337:refnum<vi>, error out=w336:errorcluster)  [unwired: 3 in, 3 out]
                    n255 = invoke class="VI" method="FP.Open"(reference=w337, error in=w336, "Activate"=TRUE ("Activate?")) -> (error out=w335:errorcluster)  [unwired: 2 in, 4 out]
                    n256 = vi-ref "Checkers PvP With File Loading.vi"() -> (w334:refnum<vi>)
                    n257 = invoke class="VI" method="Abort VI"(reference=w334, error in=w335) -> ()  [unwired: 1 in, 3 out]
                  }
                  frame True {
                    n258 = vi-ref "Checkers New Game.vi"() -> (w348:refnum<vi>)
                    n259 = vi-ref "Checkers Gymnopedie Music Player.vi"() -> (w339:refnum<vi>)
                    n260 = invoke class="VI" method="Run VI"(reference=w339, "Wait until done"=FALSE ("Wait Until Done")) -> ()  [unwired: 3 in, 5 out]
                    n261 = invoke class="VI" method="Run VI"(reference=w348, "Wait until done"=FALSE ("Wait Until Done")) -> (reference out=w347:refnum<vi>, error out=w346:errorcluster)  [unwired: 3 in, 3 out]
                    n262 = vi-ref "Checkers Palladio Music Player.vi"() -> (w341:refnum<vi>)
                    n263 = invoke class="VI" method="FP.Open"(reference=w347, error in=w346, "Activate"=TRUE ("Activate?")) -> (error out=w345:errorcluster)  [unwired: 2 in, 4 out]
                    n264 = vi-ref "Checkers PvP With File Loading.vi"() -> (w344:refnum<vi>)
                    n265 = invoke class="VI" method="Abort VI"(reference=w341) -> ()  [unwired: 2 in, 3 out]
                    n266 = invoke class="VI" method="Abort VI"(reference=w344, error in=w345) -> ()  [unwired: 1 in, 3 out]
                  }
                }
              }
              frame True {
                n267 = local read "Player 2 Name"() -> (w349:string)
                n268 = Format Into String(format string="GAME OVER. %s WINS!", w349) -> (resulting string=w353:string)  [unwired: 2 in, 1 out]
                n269 = local write "Game String"(w353) -> ()
                n270 = Two Button Dialog(message=w353, 1:"Main Menu" ("F button name (\"Cancel\")"), 2:"New Game" ("T button name (\"OK\")")) -> (T button?=w350:bool)
                n271 = case shown="True" w350 {
                  frame False {
                    n272 = vi-ref "Checkers Main Menu.vi"() -> (w361:refnum<vi>)
                    n273 = invoke class="VI" method="Run VI"(reference=w361, "Wait until done"=FALSE ("Wait Until Done")) -> (reference out=w360:refnum<vi>, error out=w359:errorcluster)  [unwired: 3 in, 3 out]
                    n274 = invoke class="VI" method="FP.Open"(reference=w360, error in=w359, "Activate"=TRUE ("Activate?")) -> (error out=w358:errorcluster)  [unwired: 2 in, 4 out]
                    n275 = vi-ref "Checkers PvP With File Loading.vi"() -> (w357:refnum<vi>)
                    n276 = invoke class="VI" method="Abort VI"(reference=w357, error in=w358) -> ()  [unwired: 1 in, 3 out]
                  }
                  frame True {
                    n277 = vi-ref "Checkers New Game.vi"() -> (w371:refnum<vi>)
                    n278 = vi-ref "Checkers Gymnopedie Music Player.vi"() -> (w362:refnum<vi>)
                    n279 = invoke class="VI" method="Run VI"(reference=w371, "Wait until done"=FALSE ("Wait Until Done")) -> (reference out=w370:refnum<vi>, error out=w369:errorcluster)  [unwired: 3 in, 3 out]
                    n280 = invoke class="VI" method="Run VI"(reference=w362, "Wait until done"=FALSE ("Wait Until Done")) -> ()  [unwired: 3 in, 5 out]
                    n281 = vi-ref "Checkers Palladio Music Player.vi"() -> (w364:refnum<vi>)
                    n282 = invoke class="VI" method="FP.Open"(reference=w370, error in=w369, "Activate"=TRUE ("Activate?")) -> (error out=w368:errorcluster)  [unwired: 2 in, 4 out]
                    n283 = vi-ref "Checkers PvP With File Loading.vi"() -> (w367:refnum<vi>)
                    n284 = invoke class="VI" method="Abort VI"(reference=w364) -> ()  [unwired: 2 in, 3 out]
                    n285 = invoke class="VI" method="Abort VI"(reference=w367, error in=w368) -> ()  [unwired: 1 in, 3 out]
                  }
                }
              }
            }
          }
        }
      }
      event "Save": Value Change {
        n286 = event-data() -> ()  [unwired: 1 in, 6 out]
        n287 = global read "Game Info Global Variable.vi" "P1 King Text Green Color"() -> (w431:i32)
        n288 = global read "Game Info Global Variable.vi" "P2 King Text Green Color"() -> (w425:i32)
        n289 = global read "Game Info Global Variable.vi" "P1 King Text Blue Color"() -> (w430:i32)
        n290 = global read "Game Info Global Variable.vi" "P2 King Text Blue Color"() -> (w424:i32)
        n291 = global read "Game Info Global Variable.vi" "P1 King Text Red Color"() -> (w432:i32)
        n292 = global read "Game Info Global Variable.vi" "P2 King Text Red Color"() -> (w426:i32)
        n293 = global read "Game Info Global Variable.vi" "P1 Green Color"() -> (w434:i32)
        n294 = global read "Game Info Global Variable.vi" "P2 Green Color"() -> (w428:i32)
        n295 = local read "Player 1 Name"() -> (w438:string)
        n296 = local read "Player 2 Name"() -> (w437:string)
        n297 = global read "Game Info Global Variable.vi" "P1 Red Color"() -> (w435:i32)
        n298 = global read "Game Info Global Variable.vi" "P1 Blue Color"() -> (w433:i32)
        n299 = global read "Game Info Global Variable.vi" "P2 Blue Color"() -> (w427:i32)
        n300 = global read "Game Info Global Variable.vi" "P2 Red Color"() -> (w429:i32)
        n301 = Format Into String(w438, w437, w435, w434, w433, w432, w431, w430, w429, w428, w427, w426, w425, w424) -> (resulting string=w436:refnum<file>)  [unwired: 3 in, 1 out]
        n302 = stacked-sequence {
          tunnel: [w439 _ _ _ _ _ _ _ _ _ _ _ _ _ _ _ _ _ _ _ _ _ _ _ _ _ _ _ _ _ _ _ _ _ _ _ _ _ _ _ _ _ _ _ _ _ _ _] -> w423
          tunnel: [_ w440 _ _ _ _ _ _ _ _ _ _ _ _ _ _ _ _ _ _ _ _ _ _ _ _ _ _ _ _ _ _ _ _ _ _ _ _ _ _ _ _ _ _ _ _ _ _] -> w422
          tunnel: [_ _ w441 _ _ _ _ _ _ _ _ _ _ _ _ _ _ _ _ _ _ _ _ _ _ _ _ _ _ _ _ _ _ _ _ _ _ _ _ _ _ _ _ _ _ _ _ _] -> w421
          tunnel: [_ _ _ w442 _ _ _ _ _ _ _ _ _ _ _ _ _ _ _ _ _ _ _ _ _ _ _ _ _ _ _ _ _ _ _ _ _ _ _ _ _ _ _ _ _ _ _ _] -> w420
          tunnel: [_ _ _ _ w443 _ _ _ _ _ _ _ _ _ _ _ _ _ _ _ _ _ _ _ _ _ _ _ _ _ _ _ _ _ _ _ _ _ _ _ _ _ _ _ _ _ _ _] -> w419
          tunnel: [_ _ _ _ _ w444 _ _ _ _ _ _ _ _ _ _ _ _ _ _ _ _ _ _ _ _ _ _ _ _ _ _ _ _ _ _ _ _ _ _ _ _ _ _ _ _ _ _] -> w418
          tunnel: [_ _ _ _ _ _ w445 _ _ _ _ _ _ _ _ _ _ _ _ _ _ _ _ _ _ _ _ _ _ _ _ _ _ _ _ _ _ _ _ _ _ _ _ _ _ _ _ _] -> w417
          tunnel: [_ _ _ _ _ _ _ w446 _ _ _ _ _ _ _ _ _ _ _ _ _ _ _ _ _ _ _ _ _ _ _ _ _ _ _ _ _ _ _ _ _ _ _ _ _ _ _ _] -> w416
          tunnel: [_ _ _ _ _ _ _ _ w447 _ _ _ _ _ _ _ _ _ _ _ _ _ _ _ _ _ _ _ _ _ _ _ _ _ _ _ _ _ _ _ _ _ _ _ _ _ _ _] -> w415
          tunnel: [_ _ _ _ _ _ _ _ _ w448 _ _ _ _ _ _ _ _ _ _ _ _ _ _ _ _ _ _ _ _ _ _ _ _ _ _ _ _ _ _ _ _ _ _ _ _ _ _] -> w414
          tunnel: [_ _ _ _ _ _ _ _ _ _ w449 _ _ _ _ _ _ _ _ _ _ _ _ _ _ _ _ _ _ _ _ _ _ _ _ _ _ _ _ _ _ _ _ _ _ _ _ _] -> w413
          tunnel: [_ _ _ _ _ _ _ _ _ _ _ w450 _ _ _ _ _ _ _ _ _ _ _ _ _ _ _ _ _ _ _ _ _ _ _ _ _ _ _ _ _ _ _ _ _ _ _ _] -> w412
          tunnel: [_ _ _ _ _ _ _ _ _ _ _ _ w451 _ _ _ _ _ _ _ _ _ _ _ _ _ _ _ _ _ _ _ _ _ _ _ _ _ _ _ _ _ _ _ _ _ _ _] -> w410
          tunnel: [_ _ _ _ _ _ _ _ _ _ _ _ _ w452 _ _ _ _ _ _ _ _ _ _ _ _ _ _ _ _ _ _ _ _ _ _ _ _ _ _ _ _ _ _ _ _ _ _] -> w409
          tunnel: [_ _ _ _ _ _ _ _ _ _ _ _ _ _ w453 _ _ _ _ _ _ _ _ _ _ _ _ _ _ _ _ _ _ _ _ _ _ _ _ _ _ _ _ _ _ _ _ _] -> w408
          tunnel: [_ _ _ _ _ _ _ _ _ _ _ _ _ _ _ w454 _ _ _ _ _ _ _ _ _ _ _ _ _ _ _ _ _ _ _ _ _ _ _ _ _ _ _ _ _ _ _ _] -> w407
          tunnel: [_ _ _ _ _ _ _ _ _ _ _ _ _ _ _ _ w455 _ _ _ _ _ _ _ _ _ _ _ _ _ _ _ _ _ _ _ _ _ _ _ _ _ _ _ _ _ _ _] -> w406
          tunnel: [_ _ _ _ _ _ _ _ _ _ _ _ _ _ _ _ _ w456 _ _ _ _ _ _ _ _ _ _ _ _ _ _ _ _ _ _ _ _ _ _ _ _ _ _ _ _ _ _] -> w405
          tunnel: [_ _ _ _ _ _ _ _ _ _ _ _ _ _ _ _ _ _ w457 _ _ _ _ _ _ _ _ _ _ _ _ _ _ _ _ _ _ _ _ _ _ _ _ _ _ _ _ _] -> w404
          tunnel: [_ _ _ _ _ _ _ _ _ _ _ _ _ _ _ _ _ _ _ w458 _ _ _ _ _ _ _ _ _ _ _ _ _ _ _ _ _ _ _ _ _ _ _ _ _ _ _ _] -> w403
          tunnel: [_ _ _ _ _ _ _ _ _ _ _ _ _ _ _ _ _ _ _ _ w459 _ _ _ _ _ _ _ _ _ _ _ _ _ _ _ _ _ _ _ _ _ _ _ _ _ _ _] -> w402
          tunnel: [_ _ _ _ _ _ _ _ _ _ _ _ _ _ _ _ _ _ _ _ _ w460 _ _ _ _ _ _ _ _ _ _ _ _ _ _ _ _ _ _ _ _ _ _ _ _ _ _] -> w401
          tunnel: [_ _ _ _ _ _ _ _ _ _ _ _ _ _ _ _ _ _ _ _ _ _ w461 _ _ _ _ _ _ _ _ _ _ _ _ _ _ _ _ _ _ _ _ _ _ _ _ _] -> w400
          tunnel: [_ _ _ _ _ _ _ _ _ _ _ _ _ _ _ _ _ _ _ _ _ _ _ w462 _ _ _ _ _ _ _ _ _ _ _ _ _ _ _ _ _ _ _ _ _ _ _ _] -> w399
          tunnel: [_ _ _ _ _ _ _ _ _ _ _ _ _ _ _ _ _ _ _ _ _ _ _ _ w463 _ _ _ _ _ _ _ _ _ _ _ _ _ _ _ _ _ _ _ _ _ _ _] -> w397
          tunnel: [_ _ _ _ _ _ _ _ _ _ _ _ _ _ _ _ _ _ _ _ _ _ _ _ _ w464 _ _ _ _ _ _ _ _ _ _ _ _ _ _ _ _ _ _ _ _ _ _] -> w396
          tunnel: [_ _ _ _ _ _ _ _ _ _ _ _ _ _ _ _ _ _ _ _ _ _ _ _ _ _ w465 _ _ _ _ _ _ _ _ _ _ _ _ _ _ _ _ _ _ _ _ _] -> w395
          tunnel: [_ _ _ _ _ _ _ _ _ _ _ _ _ _ _ _ _ _ _ _ _ _ _ _ _ _ _ w466 _ _ _ _ _ _ _ _ _ _ _ _ _ _ _ _ _ _ _ _] -> w394
          tunnel: [_ _ _ _ _ _ _ _ _ _ _ _ _ _ _ _ _ _ _ _ _ _ _ _ _ _ _ _ w467 _ _ _ _ _ _ _ _ _ _ _ _ _ _ _ _ _ _ _] -> w393
          tunnel: [_ _ _ _ _ _ _ _ _ _ _ _ _ _ _ _ _ _ _ _ _ _ _ _ _ _ _ _ _ w468 _ _ _ _ _ _ _ _ _ _ _ _ _ _ _ _ _ _] -> w392
          tunnel: [_ _ _ _ _ _ _ _ _ _ _ _ _ _ _ _ _ _ _ _ _ _ _ _ _ _ _ _ _ _ w469 _ _ _ _ _ _ _ _ _ _ _ _ _ _ _ _ _] -> w391
          tunnel: [_ _ _ _ _ _ _ _ _ _ _ _ _ _ _ _ _ _ _ _ _ _ _ _ _ _ _ _ _ _ _ w470 _ _ _ _ _ _ _ _ _ _ _ _ _ _ _ _] -> w390
          tunnel: [_ _ _ _ _ _ _ _ _ _ _ _ _ _ _ _ _ _ _ _ _ _ _ _ _ _ _ _ _ _ _ _ w471 _ _ _ _ _ _ _ _ _ _ _ _ _ _ _] -> w389
          tunnel: [_ _ _ _ _ _ _ _ _ _ _ _ _ _ _ _ _ _ _ _ _ _ _ _ _ _ _ _ _ _ _ _ _ w472 _ _ _ _ _ _ _ _ _ _ _ _ _ _] -> w388
          tunnel: [_ _ _ _ _ _ _ _ _ _ _ _ _ _ _ _ _ _ _ _ _ _ _ _ _ _ _ _ _ _ _ _ _ _ w473 _ _ _ _ _ _ _ _ _ _ _ _ _] -> w387
          tunnel: [_ _ _ _ _ _ _ _ _ _ _ _ _ _ _ _ _ _ _ _ _ _ _ _ _ _ _ _ _ _ _ _ _ _ _ w474 _ _ _ _ _ _ _ _ _ _ _ _] -> w386
          tunnel: [_ _ _ _ _ _ _ _ _ _ _ _ _ _ _ _ _ _ _ _ _ _ _ _ _ _ _ _ _ _ _ _ _ _ _ _ w475 _ _ _ _ _ _ _ _ _ _ _] -> w384
          tunnel: [_ _ _ _ _ _ _ _ _ _ _ _ _ _ _ _ _ _ _ _ _ _ _ _ _ _ _ _ _ _ _ _ _ _ _ _ _ w476 _ _ _ _ _ _ _ _ _ _] -> w383
          tunnel: [_ _ _ _ _ _ _ _ _ _ _ _ _ _ _ _ _ _ _ _ _ _ _ _ _ _ _ _ _ _ _ _ _ _ _ _ _ _ w477 _ _ _ _ _ _ _ _ _] -> w382
          tunnel: [_ _ _ _ _ _ _ _ _ _ _ _ _ _ _ _ _ _ _ _ _ _ _ _ _ _ _ _ _ _ _ _ _ _ _ _ _ _ _ w478 _ _ _ _ _ _ _ _] -> w381
          tunnel: [_ _ _ _ _ _ _ _ _ _ _ _ _ _ _ _ _ _ _ _ _ _ _ _ _ _ _ _ _ _ _ _ _ _ _ _ _ _ _ _ w479 _ _ _ _ _ _ _] -> w380
          tunnel: [_ _ _ _ _ _ _ _ _ _ _ _ _ _ _ _ _ _ _ _ _ _ _ _ _ _ _ _ _ _ _ _ _ _ _ _ _ _ _ _ _ w480 _ _ _ _ _ _] -> w379
          tunnel: [_ _ _ _ _ _ _ _ _ _ _ _ _ _ _ _ _ _ _ _ _ _ _ _ _ _ _ _ _ _ _ _ _ _ _ _ _ _ _ _ _ _ w481 _ _ _ _ _] -> w378
          tunnel: [_ _ _ _ _ _ _ _ _ _ _ _ _ _ _ _ _ _ _ _ _ _ _ _ _ _ _ _ _ _ _ _ _ _ _ _ _ _ _ _ _ _ _ w482 _ _ _ _] -> w377
          tunnel: [_ _ _ _ _ _ _ _ _ _ _ _ _ _ _ _ _ _ _ _ _ _ _ _ _ _ _ _ _ _ _ _ _ _ _ _ _ _ _ _ _ _ _ _ w483 _ _ _] -> w376
          tunnel: [_ _ _ _ _ _ _ _ _ _ _ _ _ _ _ _ _ _ _ _ _ _ _ _ _ _ _ _ _ _ _ _ _ _ _ _ _ _ _ _ _ _ _ _ _ w484 _ _] -> w375
          tunnel: [_ _ _ _ _ _ _ _ _ _ _ _ _ _ _ _ _ _ _ _ _ _ _ _ _ _ _ _ _ _ _ _ _ _ _ _ _ _ _ _ _ _ _ _ _ _ w485 _] -> w374
          tunnel: [_ _ _ _ _ _ _ _ _ _ _ _ _ _ _ _ _ _ _ _ _ _ _ _ _ _ _ _ _ _ _ _ _ _ _ _ _ _ _ _ _ _ _ _ _ _ _ w486] -> w373
          frame #0 {
            n303 = property on="P1 Piece" class="Pict"() -> ("Position"=w439:T1)  [unwired: 2 in, 2 out]
          }
          frame #1 {
            n304 = property on="P1 Piece 2" class="Pict"() -> ("Position"=w440:T1)  [unwired: 2 in, 2 out]
          }
          frame #2 {
            n305 = property on="P1 Piece 3" class="Pict"() -> ("Position"=w441:T1)  [unwired: 2 in, 2 out]
          }
          frame #3 {
            n306 = property on="P1 Piece 4" class="Pict"() -> ("Position"=w442:T1)  [unwired: 2 in, 2 out]
          }
          frame #4 {
            n307 = property on="P1 Piece 5" class="Pict"() -> ("Position"=w443:T1)  [unwired: 2 in, 2 out]
          }
          frame #5 {
            n308 = property on="P1 Piece 6" class="Pict"() -> ("Position"=w444:T1)  [unwired: 2 in, 2 out]
          }
          frame #6 {
            n309 = property on="P1 Piece 7" class="Pict"() -> ("Position"=w445:T1)  [unwired: 2 in, 2 out]
          }
          frame #7 {
            n310 = property on="P1 Piece 8" class="Pict"() -> ("Position"=w446:T1)  [unwired: 2 in, 2 out]
          }
          frame #8 {
            n311 = property on="P1 Piece 9" class="Pict"() -> ("Position"=w447:T1)  [unwired: 2 in, 2 out]
          }
          frame #9 {
            n312 = property on="P1 Piece 10" class="Pict"() -> ("Position"=w448:T1)  [unwired: 2 in, 2 out]
          }
          frame #10 {
            n313 = property on="P1 Piece 11" class="Pict"() -> ("Position"=w449:T1)  [unwired: 2 in, 2 out]
          }
          frame #11 {
            n314 = property on="P1 Piece 12" class="Pict"() -> ("Position"=w450:T1)  [unwired: 2 in, 2 out]
          }
          frame #12 {
            n315 = property on="P2 Piece" class="Pict"() -> ("Position"=w451:T1)  [unwired: 2 in, 2 out]
          }
          frame #13 {
            n316 = property on="P2 Piece 2" class="Pict"() -> ("Position"=w452:T1)  [unwired: 2 in, 2 out]
          }
          frame #14 {
            n317 = property on="P2 Piece 3" class="Pict"() -> ("Position"=w453:T1)  [unwired: 2 in, 2 out]
          }
          frame #15 {
            n318 = property on="P2 Piece 4" class="Pict"() -> ("Position"=w454:T1)  [unwired: 2 in, 2 out]
          }
          frame #16 {
            n319 = property on="P2 Piece 5" class="Pict"() -> ("Position"=w455:T1)  [unwired: 2 in, 2 out]
          }
          frame #17 {
            n320 = property on="P2 Piece 6" class="Pict"() -> ("Position"=w456:T1)  [unwired: 2 in, 2 out]
          }
          frame #18 {
            n321 = property on="P2 Piece 7" class="Pict"() -> ("Position"=w457:T1)  [unwired: 2 in, 2 out]
          }
          frame #19 {
            n322 = property on="P2 Piece 8" class="Pict"() -> ("Position"=w458:T1)  [unwired: 2 in, 2 out]
          }
          frame #20 {
            n323 = property on="P2 Piece 9" class="Pict"() -> ("Position"=w459:T1)  [unwired: 2 in, 2 out]
          }
          frame #21 {
            n324 = property on="P2 Piece 10" class="Pict"() -> ("Position"=w460:T1)  [unwired: 2 in, 2 out]
          }
          frame #22 {
            n325 = property on="P2 Piece 11" class="Pict"() -> ("Position"=w461:T1)  [unwired: 2 in, 2 out]
          }
          frame #23 {
            n326 = property on="P2 Piece 12" class="Pict"() -> ("Position"=w462:T1)  [unwired: 2 in, 2 out]
          }
          frame #24 {
            n327 = property on="P1 King" class="Pict"() -> ("Position"=w463:T1)  [unwired: 2 in, 2 out]
          }
          frame #25 {
            n328 = property on="P1 King 2" class="Pict"() -> ("Position"=w464:T1)  [unwired: 2 in, 2 out]
          }
          frame #26 {
            n329 = property on="P1 King 3" class="Pict"() -> ("Position"=w465:T1)  [unwired: 2 in, 2 out]
          }
          frame #27 {
            n330 = property on="P1 King 4" class="Pict"() -> ("Position"=w466:T1)  [unwired: 2 in, 2 out]
          }
          frame #28 {
            n331 = property on="P1 King 5" class="Pict"() -> ("Position"=w467:T1)  [unwired: 2 in, 2 out]
          }
          frame #29 {
            n332 = property on="P1 King 6" class="Pict"() -> ("Position"=w468:T1)  [unwired: 2 in, 2 out]
          }
          frame #30 {
            n333 = property on="P1 King 7" class="Pict"() -> ("Position"=w469:T1)  [unwired: 2 in, 2 out]
          }
          frame #31 {
            n334 = property on="P1 King 8" class="Pict"() -> ("Position"=w470:T1)  [unwired: 2 in, 2 out]
          }
          frame #32 {
            n335 = property on="P1 King 9" class="Pict"() -> ("Position"=w471:T1)  [unwired: 2 in, 2 out]
          }
          frame #33 {
            n336 = property on="P1 King 10" class="Pict"() -> ("Position"=w472:T1)  [unwired: 2 in, 2 out]
          }
          frame #34 {
            n337 = property on="P1 King 11" class="Pict"() -> ("Position"=w473:T1)  [unwired: 2 in, 2 out]
          }
          frame #35 {
            n338 = property on="P1 King 12" class="Pict"() -> ("Position"=w474:T1)  [unwired: 2 in, 2 out]
          }
          frame #36 {
            n339 = property on="P2 King" class="Pict"() -> ("Position"=w475:T1)  [unwired: 2 in, 2 out]
          }
          frame #37 {
            n340 = property on="P2 King 2" class="Pict"() -> ("Position"=w476:T1)  [unwired: 2 in, 2 out]
          }
          frame #38 {
            n341 = property on="P2 King 3" class="Pict"() -> ("Position"=w477:T1)  [unwired: 2 in, 2 out]
          }
          frame #39 {
            n342 = property on="P2 King 4" class="Pict"() -> ("Position"=w478:T1)  [unwired: 2 in, 2 out]
          }
          frame #40 {
            n343 = property on="P2 King 5" class="Pict"() -> ("Position"=w479:T1)  [unwired: 2 in, 2 out]
          }
          frame #41 {
            n344 = property on="P2 King 6" class="Pict"() -> ("Position"=w480:T1)  [unwired: 2 in, 2 out]
          }
          frame #42 {
            n345 = property on="P2 King 7" class="Pict"() -> ("Position"=w481:T1)  [unwired: 2 in, 2 out]
          }
          frame #43 {
            n346 = property on="P2 King 8" class="Pict"() -> ("Position"=w482:T1)  [unwired: 2 in, 2 out]
          }
          frame #44 {
            n347 = property on="P2 King 9" class="Pict"() -> ("Position"=w483:T1)  [unwired: 2 in, 2 out]
          }
          frame #45 {
            n348 = property on="P2 King 10" class="Pict"() -> ("Position"=w484:T1)  [unwired: 2 in, 2 out]
          }
          frame #46 {
            n349 = property on="P2 King 11" class="Pict"() -> ("Position"=w485:T1)  [unwired: 2 in, 2 out]
          }
          frame #47 {
            n350 = property on="P2 King 12" class="Pict"() -> ("Position"=w486:T1)  [unwired: 2 in, 2 out]
          }
        }
        n351 = Build Array(w423, w422, w421, w420, w419, w418, w417, w416, w415, w414, w413, w412) -> (w411:T1[])
        n352 = Build Array (concatenate)(w411, w410, w409, w408, w407, w406, w405, w404, w403, w402, w401, w400, w399) -> (w398:T1[])
        n353 = Build Array (concatenate)(w398, w397, w396, w395, w394, w393, w392, w391, w390, w389, w388, w387, w386) -> (w385:T1[])
        n354 = Build Array (concatenate)(w385, w384, w383, w382, w381, w380, w379, w378, w377, w376, w375, w374, w373) -> (w372:T1[])
        n355 = for {
          tunnel: w372 -> [w494] mode=indexing
          tunnel: w436 -> [w493]
          n356 = Unbundle(w494) -> ("Left"=w488:i32, "Top"=w487:i32)
          n357 = Set File Position(refnum=w493, from (0:start)=enum16{"start", "end", "current"}."end") -> (refnum out=w490:refnum<file>)  [unwired: 2 in, 1 out]
          n358 = Format Into String(initial string=w490, " " ("input 1")) -> (resulting string=w489:refnum<file>)  [unwired: 2 in, 1 out]
          n359 = Format Into String(initial string=w489, w488, w487) -> ()  [unwired: 2 in, 2 out]
        }
      }
      event "Save and Quit": Value Change {
        n360 = event-data() -> ()  [unwired: 1 in, 6 out]
        n361 = flat-sequence {
          tunnel: [w495] -> _
          frame #0 {
            n362 = global read "Game Info Global Variable.vi" "P1 King Text Green Color"() -> (w504:i32)
            n363 = global read "Game Info Global Variable.vi" "P2 King Text Green Color"() -> (w498:i32)
            n364 = global read "Game Info Global Variable.vi" "P1 King Text Blue Color"() -> (w503:i32)
            n365 = global read "Game Info Global Variable.vi" "P2 King Text Blue Color"() -> (w497:i32)
            n366 = global read "Game Info Global Variable.vi" "P1 King Text Red Color"() -> (w505:i32)
            n367 = global read "Game Info Global Variable.vi" "P2 King Text Red Color"() -> (w499:i32)
            n368 = global read "Game Info Global Variable.vi" "P1 Green Color"() -> (w507:i32)
            n369 = global read "Game Info Global Variable.vi" "P2 Green Color"() -> (w501:i32)
            n370 = local read "Player 1 Name"() -> (w510:string)
            n371 = local read "Player 2 Name"() -> (w509:string)
            n372 = global read "Game Info Global Variable.vi" "P1 Red Color"() -> (w508:i32)
            n373 = global read "Game Info Global Variable.vi" "P1 Blue Color"() -> (w506:i32)
            n374 = global read "Game Info Global Variable.vi" "P2 Blue Color"() -> (w500:i32)
            n375 = global read "Game Info Global Variable.vi" "P2 Red Color"() -> (w502:i32)
            n376 = Format Into String(w510, w509, w508, w507, w506, w505, w504, w503, w502, w501, w500, w499, w498, w497) -> (resulting string=w496:refnum<file>)  [unwired: 3 in, 1 out]
            n377 = stacked-sequence {
              tunnel: [w562 _ _ _ _ _ _ _ _ _ _ _ _ _ _ _ _ _ _ _ _ _ _ _ _ _ _ _ _ _ _ _ _ _ _ _ _ _ _ _ _ _ _ _ _ _ _ _] -> w511
              tunnel: [_ w563 _ _ _ _ _ _ _ _ _ _ _ _ _ _ _ _ _ _ _ _ _ _ _ _ _ _ _ _ _ _ _ _ _ _ _ _ _ _ _ _ _ _ _ _ _ _] -> w512
              tunnel: [_ _ w564 _ _ _ _ _ _ _ _ _ _ _ _ _ _ _ _ _ _ _ _ _ _ _ _ _ _ _ _ _ _ _ _ _ _ _ _ _ _ _ _ _ _ _ _ _] -> w513
              tunnel: [_ _ _ w565 _ _ _ _ _ _ _ _ _ _ _ _ _ _ _ _ _ _ _ _ _ _ _ _ _ _ _ _ _ _ _ _ _ _ _ _ _ _ _ _ _ _ _ _] -> w514
              tunnel: [_ _ _ _ w566 _ _ _ _ _ _ _ _ _ _ _ _ _ _ _ _ _ _ _ _ _ _ _ _ _ _ _ _ _ _ _ _ _ _ _ _ _ _ _ _ _ _ _] -> w515
              tunnel: [_ _ _ _ _ w567 _ _ _ _ _ _ _ _ _ _ _ _ _ _ _ _ _ _ _ _ _ _ _ _ _ _ _ _ _ _ _ _ _ _ _ _ _ _ _ _ _ _] -> w516
              tunnel: [_ _ _ _ _ _ w568 _ _ _ _ _ _ _ _ _ _ _ _ _ _ _ _ _ _ _ _ _ _ _ _ _ _ _ _ _ _ _ _ _ _ _ _ _ _ _ _ _] -> w517
              tunnel: [_ _ _ _ _ _ _ w569 _ _ _ _ _ _ _ _ _ _ _ _ _ _ _ _ _ _ _ _ _ _ _ _ _ _ _ _ _ _ _ _ _ _ _ _ _ _ _ _] -> w518
              tunnel: [_ _ _ _ _ _ _ _ w570 _ _ _ _ _ _ _ _ _ _ _ _ _ _ _ _ _ _ _ _ _ _ _ _ _ _ _ _ _ _ _ _ _ _ _ _ _ _ _] -> w519
              tunnel: [_ _ _ _ _ _ _ _ _ w571 _ _ _ _ _ _ _ _ _ _ _ _ _ _ _ _ _ _ _ _ _ _ _ _ _ _ _ _ _ _ _ _ _ _ _ _ _ _] -> w520
              tunnel: [_ _ _ _ _ _ _ _ _ _ w572 _ _ _ _ _ _ _ _ _ _ _ _ _ _ _ _ _ _ _ _ _ _ _ _ _ _ _ _ _ _ _ _ _ _ _ _ _] -> w521
              tunnel: [_ _ _ _ _ _ _ _ _ _ _ w573 _ _ _ _ _ _ _ _ _ _ _ _ _ _ _ _ _ _ _ _ _ _ _ _ _ _ _ _ _ _ _ _ _ _ _ _] -> w522
              tunnel: [_ _ _ _ _ _ _ _ _ _ _ _ w574 _ _ _ _ _ _ _ _ _ _ _ _ _ _ _ _ _ _ _ _ _ _ _ _ _ _ _ _ _ _ _ _ _ _ _] -> w524
              tunnel: [_ _ _ _ _ _ _ _ _ _ _ _ _ w575 _ _ _ _ _ _ _ _ _ _ _ _ _ _ _ _ _ _ _ _ _ _ _ _ _ _ _ _ _ _ _ _ _ _] -> w525
              tunnel: [_ _ _ _ _ _ _ _ _ _ _ _ _ _ w576 _ _ _ _ _ _ _ _ _ _ _ _ _ _ _ _ _ _ _ _ _ _ _ _ _ _ _ _ _ _ _ _ _] -> w526
              tunnel: [_ _ _ _ _ _ _ _ _ _ _ _ _ _ _ w577 _ _ _ _ _ _ _ _ _ _ _ _ _ _ _ _ _ _ _ _ _ _ _ _ _ _ _ _ _ _ _ _] -> w527
              tunnel: [_ _ _ _ _ _ _ _ _ _ _ _ _ _ _ _ w578 _ _ _ _ _ _ _ _ _ _ _ _ _ _ _ _ _ _ _ _ _ _ _ _ _ _ _ _ _ _ _] -> w528
              tunnel: [_ _ _ _ _ _ _ _ _ _ _ _ _ _ _ _ _ w579 _ _ _ _ _ _ _ _ _ _ _ _ _ _ _ _ _ _ _ _ _ _ _ _ _ _ _ _ _ _] -> w529
              tunnel: [_ _ _ _ _ _ _ _ _ _ _ _ _ _ _ _ _ _ w580 _ _ _ _ _ _ _ _ _ _ _ _ _ _ _ _ _ _ _ _ _ _ _ _ _ _ _ _ _] -> w530
              tunnel: [_ _ _ _ _ _ _ _ _ _ _ _ _ _ _ _ _ _ _ w581 _ _ _ _ _ _ _ _ _ _ _ _ _ _ _ _ _ _ _ _ _ _ _ _ _ _ _ _] -> w531
              tunnel: [_ _ _ _ _ _ _ _ _ _ _ _ _ _ _ _ _ _ _ _ w582 _ _ _ _ _ _ _ _ _ _ _ _ _ _ _ _ _ _ _ _ _ _ _ _ _ _ _] -> w532
              tunnel: [_ _ _ _ _ _ _ _ _ _ _ _ _ _ _ _ _ _ _ _ _ w583 _ _ _ _ _ _ _ _ _ _ _ _ _ _ _ _ _ _ _ _ _ _ _ _ _ _] -> w533
              tunnel: [_ _ _ _ _ _ _ _ _ _ _ _ _ _ _ _ _ _ _ _ _ _ w584 _ _ _ _ _ _ _ _ _ _ _ _ _ _ _ _ _ _ _ _ _ _ _ _ _] -> w535
              tunnel: [_ _ _ _ _ _ _ _ _ _ _ _ _ _ _ _ _ _ _ _ _ _ _ w585 _ _ _ _ _ _ _ _ _ _ _ _ _ _ _ _ _ _ _ _ _ _ _ _] -> w534
              tunnel: [_ _ _ _ _ _ _ _ _ _ _ _ _ _ _ _ _ _ _ _ _ _ _ _ w586 _ _ _ _ _ _ _ _ _ _ _ _ _ _ _ _ _ _ _ _ _ _ _] -> w538
              tunnel: [_ _ _ _ _ _ _ _ _ _ _ _ _ _ _ _ _ _ _ _ _ _ _ _ _ w587 _ _ _ _ _ _ _ _ _ _ _ _ _ _ _ _ _ _ _ _ _ _] -> w539
              tunnel: [_ _ _ _ _ _ _ _ _ _ _ _ _ _ _ _ _ _ _ _ _ _ _ _ _ _ w588 _ _ _ _ _ _ _ _ _ _ _ _ _ _ _ _ _ _ _ _ _] -> w540
              tunnel: [_ _ _ _ _ _ _ _ _ _ _ _ _ _ _ _ _ _ _ _ _ _ _ _ _ _ _ w589 _ _ _ _ _ _ _ _ _ _ _ _ _ _ _ _ _ _ _ _] -> w541
              tunnel: [_ _ _ _ _ _ _ _ _ _ _ _ _ _ _ _ _ _ _ _ _ _ _ _ _ _ _ _ w590 _ _ _ _ _ _ _ _ _ _ _ _ _ _ _ _ _ _ _] -> w542
              tunnel: [_ _ _ _ _ _ _ _ _ _ _ _ _ _ _ _ _ _ _ _ _ _ _ _ _ _ _ _ _ w591 _ _ _ _ _ _ _ _ _ _ _ _ _ _ _ _ _ _] -> w543
              tunnel: [_ _ _ _ _ _ _ _ _ _ _ _ _ _ _ _ _ _ _ _ _ _ _ _ _ _ _ _ _ _ w592 _ _ _ _ _ _ _ _ _ _ _ _ _ _ _ _ _] -> w544
              tunnel: [_ _ _ _ _ _ _ _ _ _ _ _ _ _ _ _ _ _ _ _ _ _ _ _ _ _ _ _ _ _ _ w593 _ _ _ _ _ _ _ _ _ _ _ _ _ _ _ _] -> w545
              tunnel: [_ _ _ _ _ _ _ _ _ _ _ _ _ _ _ _ _ _ _ _ _ _ _ _ _ _ _ _ _ _ _ _ w594 _ _ _ _ _ _ _ _ _ _ _ _ _ _ _] -> w546
              tunnel: [_ _ _ _ _ _ _ _ _ _ _ _ _ _ _ _ _ _ _ _ _ _ _ _ _ _ _ _ _ _ _ _ _ w595 _ _ _ _ _ _ _ _ _ _ _ _ _ _] -> w547
              tunnel: [_ _ _ _ _ _ _ _ _ _ _ _ _ _ _ _ _ _ _ _ _ _ _ _ _ _ _ _ _ _ _ _ _ _ w596 _ _ _ _ _ _ _ _ _ _ _ _ _] -> w548
              tunnel: [_ _ _ _ _ _ _ _ _ _ _ _ _ _ _ _ _ _ _ _ _ _ _ _ _ _ _ _ _ _ _ _ _ _ _ w597 _ _ _ _ _ _ _ _ _ _ _ _] -> w549
              tunnel: [_ _ _ _ _ _ _ _ _ _ _ _ _ _ _ _ _ _ _ _ _ _ _ _ _ _ _ _ _ _ _ _ _ _ _ _ w598 _ _ _ _ _ _ _ _ _ _ _] -> w550
              tunnel: [_ _ _ _ _ _ _ _ _ _ _ _ _ _ _ _ _ _ _ _ _ _ _ _ _ _ _ _ _ _ _ _ _ _ _ _ _ w599 _ _ _ _ _ _ _ _ _ _] -> w551
              tunnel: [_ _ _ _ _ _ _ _ _ _ _ _ _ _ _ _ _ _ _ _ _ _ _ _ _ _ _ _ _ _ _ _ _ _ _ _ _ _ w600 _ _ _ _ _ _ _ _ _] -> w552
              tunnel: [_ _ _ _ _ _ _ _ _ _ _ _ _ _ _ _ _ _ _ _ _ _ _ _ _ _ _ _ _ _ _ _ _ _ _ _ _ _ _ w601 _ _ _ _ _ _ _ _] -> w553
              tunnel: [_ _ _ _ _ _ _ _ _ _ _ _ _ _ _ _ _ _ _ _ _ _ _ _ _ _ _ _ _ _ _ _ _ _ _ _ _ _ _ _ w602 _ _ _ _ _ _ _] -> w554
              tunnel: [_ _ _ _ _ _ _ _ _ _ _ _ _ _ _ _ _ _ _ _ _ _ _ _ _ _ _ _ _ _ _ _ _ _ _ _ _ _ _ _ _ w603 _ _ _ _ _ _] -> w555
              tunnel: [_ _ _ _ _ _ _ _ _ _ _ _ _ _ _ _ _ _ _ _ _ _ _ _ _ _ _ _ _ _ _ _ _ _ _ _ _ _ _ _ _ _ w604 _ _ _ _ _] -> w556
              tunnel: [_ _ _ _ _ _ _ _ _ _ _ _ _ _ _ _ _ _ _ _ _ _ _ _ _ _ _ _ _ _ _ _ _ _ _ _ _ _ _ _ _ _ _ w605 _ _ _ _] -> w557
              tunnel: [_ _ _ _ _ _ _ _ _ _ _ _ _ _ _ _ _ _ _ _ _ _ _ _ _ _ _ _ _ _ _ _ _ _ _ _ _ _ _ _ _ _ _ _ w606 _ _ _] -> w558
              tunnel: [_ _ _ _ _ _ _ _ _ _ _ _ _ _ _ _ _ _ _ _ _ _ _ _ _ _ _ _ _ _ _ _ _ _ _ _ _ _ _ _ _ _ _ _ _ w607 _ _] -> w559
              tunnel: [_ _ _ _ _ _ _ _ _ _ _ _ _ _ _ _ _ _ _ _ _ _ _ _ _ _ _ _ _ _ _ _ _ _ _ _ _ _ _ _ _ _ _ _ _ _ w608 _] -> w560
              tunnel: [_ _ _ _ _ _ _ _ _ _ _ _ _ _ _ _ _ _ _ _ _ _ _ _ _ _ _ _ _ _ _ _ _ _ _ _ _ _ _ _ _ _ _ _ _ _ _ w609] -> w561
              frame #0 {
                n378 = property on="P1 Piece" class="Pict"() -> ("Position"=w562:T1)  [unwired: 2 in, 2 out]
              }
              frame #1 {
                n379 = property on="P1 Piece 2" class="Pict"() -> ("Position"=w563:T1)  [unwired: 2 in, 2 out]
              }
              frame #2 {
                n380 = property on="P1 Piece 3" class="Pict"() -> ("Position"=w564:T1)  [unwired: 2 in, 2 out]
              }
              frame #3 {
                n381 = property on="P1 Piece 4" class="Pict"() -> ("Position"=w565:T1)  [unwired: 2 in, 2 out]
              }
              frame #4 {
                n382 = property on="P1 Piece 5" class="Pict"() -> ("Position"=w566:T1)  [unwired: 2 in, 2 out]
              }
              frame #5 {
                n383 = property on="P1 Piece 6" class="Pict"() -> ("Position"=w567:T1)  [unwired: 2 in, 2 out]
              }
              frame #6 {
                n384 = property on="P1 Piece 7" class="Pict"() -> ("Position"=w568:T1)  [unwired: 2 in, 2 out]
              }
              frame #7 {
                n385 = property on="P1 Piece 8" class="Pict"() -> ("Position"=w569:T1)  [unwired: 2 in, 2 out]
              }
              frame #8 {
                n386 = property on="P1 Piece 9" class="Pict"() -> ("Position"=w570:T1)  [unwired: 2 in, 2 out]
              }
              frame #9 {
                n387 = property on="P1 Piece 10" class="Pict"() -> ("Position"=w571:T1)  [unwired: 2 in, 2 out]
              }
              frame #10 {
                n388 = property on="P1 Piece 11" class="Pict"() -> ("Position"=w572:T1)  [unwired: 2 in, 2 out]
              }
              frame #11 {
                n389 = property on="P1 Piece 12" class="Pict"() -> ("Position"=w573:T1)  [unwired: 2 in, 2 out]
              }
              frame #12 {
                n390 = property on="P2 Piece" class="Pict"() -> ("Position"=w574:T1)  [unwired: 2 in, 2 out]
              }
              frame #13 {
                n391 = property on="P2 Piece 2" class="Pict"() -> ("Position"=w575:T1)  [unwired: 2 in, 2 out]
              }
              frame #14 {
                n392 = property on="P2 Piece 3" class="Pict"() -> ("Position"=w576:T1)  [unwired: 2 in, 2 out]
              }
              frame #15 {
                n393 = property on="P2 Piece 4" class="Pict"() -> ("Position"=w577:T1)  [unwired: 2 in, 2 out]
              }
              frame #16 {
                n394 = property on="P2 Piece 5" class="Pict"() -> ("Position"=w578:T1)  [unwired: 2 in, 2 out]
              }
              frame #17 {
                n395 = property on="P2 Piece 6" class="Pict"() -> ("Position"=w579:T1)  [unwired: 2 in, 2 out]
              }
              frame #18 {
                n396 = property on="P2 Piece 7" class="Pict"() -> ("Position"=w580:T1)  [unwired: 2 in, 2 out]
              }
              frame #19 {
                n397 = property on="P2 Piece 8" class="Pict"() -> ("Position"=w581:T1)  [unwired: 2 in, 2 out]
              }
              frame #20 {
                n398 = property on="P2 Piece 9" class="Pict"() -> ("Position"=w582:T1)  [unwired: 2 in, 2 out]
              }
              frame #21 {
                n399 = property on="P2 Piece 10" class="Pict"() -> ("Position"=w583:T1)  [unwired: 2 in, 2 out]
              }
              frame #22 {
                n400 = property on="P2 Piece 11" class="Pict"() -> ("Position"=w584:T1)  [unwired: 2 in, 2 out]
              }
              frame #23 {
                n401 = property on="P2 Piece 12" class="Pict"() -> ("Position"=w585:T1)  [unwired: 2 in, 2 out]
              }
              frame #24 {
                n402 = property on="P1 King" class="Pict"() -> ("Position"=w586:T1)  [unwired: 2 in, 2 out]
              }
              frame #25 {
                n403 = property on="P1 King 2" class="Pict"() -> ("Position"=w587:T1)  [unwired: 2 in, 2 out]
              }
              frame #26 {
                n404 = property on="P1 King 3" class="Pict"() -> ("Position"=w588:T1)  [unwired: 2 in, 2 out]
              }
              frame #27 {
                n405 = property on="P1 King 4" class="Pict"() -> ("Position"=w589:T1)  [unwired: 2 in, 2 out]
              }
              frame #28 {
                n406 = property on="P1 King 5" class="Pict"() -> ("Position"=w590:T1)  [unwired: 2 in, 2 out]
              }
              frame #29 {
                n407 = property on="P1 King 6" class="Pict"() -> ("Position"=w591:T1)  [unwired: 2 in, 2 out]
              }
              frame #30 {
                n408 = property on="P1 King 7" class="Pict"() -> ("Position"=w592:T1)  [unwired: 2 in, 2 out]
              }
              frame #31 {
                n409 = property on="P1 King 8" class="Pict"() -> ("Position"=w593:T1)  [unwired: 2 in, 2 out]
              }
              frame #32 {
                n410 = property on="P1 King 9" class="Pict"() -> ("Position"=w594:T1)  [unwired: 2 in, 2 out]
              }
              frame #33 {
                n411 = property on="P1 King 10" class="Pict"() -> ("Position"=w595:T1)  [unwired: 2 in, 2 out]
              }
              frame #34 {
                n412 = property on="P1 King 11" class="Pict"() -> ("Position"=w596:T1)  [unwired: 2 in, 2 out]
              }
              frame #35 {
                n413 = property on="P1 King 12" class="Pict"() -> ("Position"=w597:T1)  [unwired: 2 in, 2 out]
              }
              frame #36 {
                n414 = property on="P2 King" class="Pict"() -> ("Position"=w598:T1)  [unwired: 2 in, 2 out]
              }
              frame #37 {
                n415 = property on="P2 King 2" class="Pict"() -> ("Position"=w599:T1)  [unwired: 2 in, 2 out]
              }
              frame #38 {
                n416 = property on="P2 King 3" class="Pict"() -> ("Position"=w600:T1)  [unwired: 2 in, 2 out]
              }
              frame #39 {
                n417 = property on="P2 King 4" class="Pict"() -> ("Position"=w601:T1)  [unwired: 2 in, 2 out]
              }
              frame #40 {
                n418 = property on="P2 King 5" class="Pict"() -> ("Position"=w602:T1)  [unwired: 2 in, 2 out]
              }
              frame #41 {
                n419 = property on="P2 King 6" class="Pict"() -> ("Position"=w603:T1)  [unwired: 2 in, 2 out]
              }
              frame #42 {
                n420 = property on="P2 King 7" class="Pict"() -> ("Position"=w604:T1)  [unwired: 2 in, 2 out]
              }
              frame #43 {
                n421 = property on="P2 King 8" class="Pict"() -> ("Position"=w605:T1)  [unwired: 2 in, 2 out]
              }
              frame #44 {
                n422 = property on="P2 King 9" class="Pict"() -> ("Position"=w606:T1)  [unwired: 2 in, 2 out]
              }
              frame #45 {
                n423 = property on="P2 King 10" class="Pict"() -> ("Position"=w607:T1)  [unwired: 2 in, 2 out]
              }
              frame #46 {
                n424 = property on="P2 King 11" class="Pict"() -> ("Position"=w608:T1)  [unwired: 2 in, 2 out]
              }
              frame #47 {
                n425 = property on="P2 King 12" class="Pict"() -> ("Position"=w609:T1)  [unwired: 2 in, 2 out]
              }
            }
            n426 = Build Array(w511, w512, w513, w514, w515, w516, w517, w518, w519, w520, w521, w522) -> (w523:T1[])
            n427 = Build Array (concatenate)(w523, w524, w525, w526, w527, w528, w529, w530, w531, w532, w533, w535, w534) -> (w536:T1[])
            n428 = Build Array (concatenate)(w536, w538, w539, w540, w541, w542, w543, w544, w545, w546, w547, w548, w549) -> (w537:T1[])
            n429 = Build Array (concatenate)(w537, w550, w551, w552, w553, w554, w555, w556, w557, w558, w559, w560, w561) -> (w495:T1[])
            n430 = for {
              tunnel: w495 -> [w617] mode=indexing
              tunnel: w496 -> [w616]
              n431 = Unbundle(w617) -> ("Left"=w611:i32, "Top"=w610:i32)
              n432 = Set File Position(refnum=w616, from (0:start)=enum16{"start", "end", "current"}."end") -> (refnum out=w613:refnum<file>)  [unwired: 2 in, 1 out]
              n433 = Format Into String(initial string=w613, " " ("input 1")) -> (resulting string=w612:refnum<file>)  [unwired: 2 in, 1 out]
              n434 = Format Into String(initial string=w612, w611, w610) -> ()  [unwired: 2 in, 2 out]
            }
          }
          frame #1 {
            n435 = vi-ref "Checkers Main Menu.vi"() -> (w621:refnum<vi>)
            n436 = vi-ref "Checkers Gymnopedie Music Player.vi"() -> (w618:refnum<vi>)
            n437 = invoke class="VI" method="Run VI"(reference=w621, "Wait until done"=FALSE ("Wait Until Done")) -> (reference out=w622:refnum<vi>, error out=w623:errorcluster)  [unwired: 3 in, 3 out]
            n438 = invoke class="VI" method="Run VI"(reference=w618, "Wait until done"=FALSE ("Wait Until Done")) -> ()  [unwired: 3 in, 5 out]
            n439 = invoke class="VI" method="FP.Open"(reference=w622, error in=w623, "Activate"=TRUE ("Activate?")) -> (error out=w624:errorcluster)  [unwired: 2 in, 4 out]
            n440 = vi-ref "Checkers Palladio Music Player.vi"() -> (w620:refnum<vi>)
            n441 = vi-ref "Checkers PvP With File Loading.vi"() -> (w625:refnum<vi>)
            n442 = invoke class="VI" method="Abort VI"(reference=w625, error in=w624) -> ()  [unwired: 1 in, 3 out]
            n443 = invoke class="VI" method="Abort VI"(reference=w620) -> ()  [unwired: 2 in, 3 out]
          }
        }
      }
      event "Quit": Value Change {
        n444 = event-data() -> ()  [unwired: 1 in, 6 out]
        n445 = Two Button Dialog(message="Are you sure you want to quit without saving?", 1:"No" ("F button name (\"Cancel\")"), 2:"Yes" ("T button name (\"OK\")")) -> (T button?=w628:bool)
        n446 = case shown="False" w628 {
          frame False {
            # "Player changed mind to quit without saving. Do nothing."
          }
          frame True {
            n447 = vi-ref "Checkers Gymnopedie Music Player.vi"() -> (w632:refnum<vi>)
            n448 = vi-ref "Checkers Main Menu.vi"() -> (w641:refnum<vi>)
            n449 = invoke class="VI" method="Run VI"(reference=w641, "Wait until done"=FALSE ("Wait Until Done")) -> (reference out=w640:refnum<vi>, error out=w639:errorcluster)  [unwired: 3 in, 3 out]
            n450 = invoke class="VI" method="Run VI"(reference=w632, "Wait until done"=FALSE ("Wait Until Done")) -> ()  [unwired: 3 in, 5 out]
            n451 = invoke class="VI" method="FP.Open"(reference=w640, error in=w639, "Activate"=TRUE ("Activate?")) -> (error out=w638:errorcluster)  [unwired: 2 in, 4 out]
            n452 = vi-ref "Checkers Palladio Music Player.vi"() -> (w634:refnum<vi>)
            n453 = vi-ref "Checkers PvP With File Loading.vi"() -> (w637:refnum<vi>)
            n454 = invoke class="VI" method="Abort VI"(reference=w637, error in=w638) -> ()  [unwired: 1 in, 3 out]
            n455 = invoke class="VI" method="Abort VI"(reference=w634) -> ()  [unwired: 2 in, 3 out]
          }
        }
      }
      event "P1 Piece", "P1 Piece 2", "P1 Piece 3", "P1 Piece 4", "P1 Piece 5", "P1 Piece 6", "P1 Piece 7", "P1 Piece 8", "P1 Piece 9", "P1 Piece 10", "P1 Piece 11", "P1 Piece 12": Mouse Down {
        n456 = event-data() -> ("CtlRef"=w647:refnum<vi>)  [unwired: 1 in, 7 out]
        n457 = local read "P1 Turn Light"() -> (w648:bool)
        n458 = case shown="True" w648 {
          tunnel: w647 -> [_ w659]
          tunnel: [_ w656] -> w646
          tunnel: [_ w654] -> w645
          tunnel: [_ w655] -> w644
          tunnel: [_ w649] -> w643
          tunnel: [_ w650] -> w642
          frame False {
            # "It's not player 1's turn yet. Do nothing."
          }
          frame True {
            # "At this point, I use an \nequation to turn the pixel\ncoordinates into the array coordinates\nof the piece that the user clicked."
            # "Left first"
            # "row[0], collumn[1]"
            n459 = property on="Property Node" class="Pict"(reference=w659) -> ("Position"=w655:T1)  [unwired: 1 in, 2 out]
            n460 = global read "Board Layout Global Variable.vi" "Board Layout"() -> (w653:dbl[][])
            n461 = Unbundle By Name(w655) -> ("Left"=w676:i32, "Top"=w674:i32)
            n462 = expression code="(x-469)/42"(w676) -> (w677:i32)
            n463 = expression code="(x-56)/42"(w674) -> (w675:i32)
            n464 = To Long Integer(number=w677) -> (32bit integer=w660:i32)
            n465 = To Long Integer(number=w675) -> (32bit integer=w661:i32)
            n466 = Build Array(w661, w660) -> (w652:i32[])
            n467 = call "MoveLogic.vi"("Array"=w653, "Coordinates"=w652) -> ("Moves"=w651:dbl[][], "Capture 1"=w650:cluster{"Left":dbl, " Top":dbl}, "Capture 2"=w649:cluster{"Left":dbl, " Top":dbl})
            n468 = Index Array(array=w651, index (row)=0) -> (element=w656:dbl[])  [unwired: 1 in]
            n469 = Index Array(array=w651, index (row)=1) -> (element=w654:dbl[])  [unwired: 1 in]
            n470 = Index Array(array=w654, index=1) -> (element=w673:dbl)
            n471 = Index Array(array=w654, index=0) -> (element=w672:dbl)
            n472 = Index Array(array=w656, index=0) -> (element=w662:dbl)
            n473 = Index Array(array=w656, index=1) -> (element=w663:dbl)
            n474 = expression code="(x*42)+56"(w672) -> (w671:dbl)
            n475 = expression code="(x*42)+469"(w673) -> (w670:dbl)
            n476 = expression code="(x*42)+56"(w662) -> (w664:dbl)
            n477 = expression code="(x*42)+469"(w663) -> (w665:dbl)
            n478 = To Long Integer(number=w670) -> (32bit integer=w669:i32)
            n479 = To Long Integer(number=w671) -> (32bit integer=w668:i32)
            n480 = To Long Integer(number=w665) -> (32bit integer=w666:i32)
            n481 = To Long Integer(number=w664) -> (32bit integer=w667:i32)
            n482 = Bundle(w669, w668) -> (w657:cluster{i32, i32})  [unwired: 1 in]
            n483 = Bundle(w666, w667) -> (w658:cluster{i32, i32})  [unwired: 1 in]
            n484 = property on="P1 Top Right Marker" class="Pict"("Position"=w657) -> ()  [unwired: 2 in, 2 out]
            n485 = property on="P1 Top Left Marker" class="Pict"("Position"=w658) -> ()  [unwired: 2 in, 2 out]
          }
        }
      }
      event "P1 King", "P1 King 2", "P1 King 3", "P1 King 4", "P1 King 5", "P1 King 6", "P1 King 7", "P1 King 8", "P1 King 9", "P1 King 10", "P1 King 11", "P1 King 12": Mouse Down {
        n486 = event-data() -> ("CtlRef"=w684:refnum<vi>)  [unwired: 1 in, 7 out]
        n487 = local read "P1 Turn Light"() -> (w685:bool)
        n488 = case shown="True" w685 {
          tunnel: w684 -> [_ w689]
          frame False {
            # "It's not player 1's turn yet. Do nothing."
          }
          frame True {
            # "At this point, I use an \nequation to turn the pixel\ncoordinates into the array coordinates\nof the piece that the user clicked."
            # "Left first"
            # "row[0], collumn[1]"
            n489 = property on="Property Node" class="Pict"(reference=w689) -> ("Position"=w690:T1)  [unwired: 1 in, 2 out]
            n490 = global read "Board Layout Global Variable.vi" "Board Layout"() -> (w688:dbl[][])
            n491 = Unbundle By Name(w690) -> ("Left"=w710:i32, "Top"=w708:i32)
            n492 = expression code="(x-469)/42"(w710) -> (w711:i32)
            n493 = expression code="(x-56)/42"(w708) -> (w709:i32)
            n494 = To Long Integer(number=w711) -> (32bit integer=w693:i32)
            n495 = To Long Integer(number=w709) -> (32bit integer=w694:i32)
            n496 = Build Array(w694, w693) -> (w686:i32[])
            n497 = call "MoveLogic.vi"("Array"=w688, "Coordinates"=w686) -> ("Moves"=w687:dbl[][])  [unwired: 2 out]
            n498 = Index Array(array=w687, index (row)=0) -> (element=w695:dbl[])  [unwired: 1 in]
            n499 = Index Array(array=w687, index (row)=1) -> (element=w714:dbl[])  [unwired: 1 in]
            n500 = Index Array(array=w714, index=1) -> (element=w707:dbl)
            n501 = Index Array(array=w714, index=0) -> (element=w706:dbl)
            n502 = Index Array(array=w695, index=0) -> (element=w696:dbl)
            n503 = Index Array(array=w695, index=1) -> (element=w697:dbl)
            n504 = expression code="(x*42)+56"(w706) -> (w705:dbl)
            n505 = expression code="(x*42)+469"(w707) -> (w704:dbl)
            n506 = expression code="(x*42)+56"(w696) -> (w698:dbl)
            n507 = expression code="(x*42)+469"(w697) -> (w699:dbl)
            n508 = To Long Integer(number=w704) -> (32bit integer=w703:i32)
            n509 = To Long Integer(number=w705) -> (32bit integer=w702:i32)
            n510 = To Long Integer(number=w699) -> (32bit integer=w700:i32)
            n511 = To Long Integer(number=w698) -> (32bit integer=w701:i32)
            n512 = Bundle(w703, w702) -> (w692:cluster{i32, i32})  [unwired: 1 in]
            n513 = Bundle(w700, w701) -> (w691:cluster{i32, i32})  [unwired: 1 in]
            n514 = property on="P1 Top Right Marker" class="Pict"("Position"=w692) -> ()  [unwired: 2 in, 2 out]
            n515 = property on="P1 Top Left Marker" class="Pict"("Position"=w691) -> ()  [unwired: 2 in, 2 out]
          }
        }
      }
      event "P2 Piece", "P2 Piece 2", "P2 Piece 3", "P2 Piece 4", "P2 Piece 5", "P2 Piece 6", "P2 Piece 7", "P2 Piece 8", "P2 Piece 9", "P2 Piece 10", "P2 Piece 11", "P2 Piece 12": Mouse Down {
        n516 = event-data() -> ("CtlRef"=w724:refnum<vi>)  [unwired: 1 in, 7 out]
        n517 = local read "P2 Turn Light"() -> (w719:bool)
        n518 = case shown="True" w719 {
          tunnel: w724 -> [_ w734]
          tunnel: [_ w729] -> w723
          tunnel: [_ w727] -> w722
          tunnel: [_ w726] -> w721
          tunnel: [_ w725] -> w720
          frame False {
            # "It's not player 1's turn yet. Do nothing."
          }
          frame True {
            # "This sub VI outputs a 2d array \nthat holds 2 coordinates indicating \nwhere the piece can go"
            # "At this point, I use an \nequation to turn the pixel\ncoordinates into the array coordinates\nof the piece that the user clicked."
            # "Left first"
            # "row[0], collumn[1]"
            n519 = property on="Property Node" class="Pict"(reference=w734) -> ("Position"=w735:T1)  [unwired: 1 in, 2 out]
            n520 = Unbundle By Name(w735) -> ("Left"=w752:i32, "Top"=w750:i32)
            n521 = global read "Board Layout Global Variable.vi" "Board Layout"() -> (w732:dbl[][])
            n522 = expression code="(x-469)/42"(w752) -> (w753:i32)
            n523 = expression code="(x-56)/42"(w750) -> (w751:i32)
            n524 = To Long Integer(number=w753) -> (32bit integer=w736:i32)
            n525 = To Long Integer(number=w751) -> (32bit integer=w737:i32)
            n526 = Build Array(w737, w736) -> (w731:i32[])
            n527 = call "MoveLogic.vi"("Array"=w732, "Coordinates"=w731) -> ("Moves"=w730:dbl[][], "Capture 1"=w725:cluster{"Left":dbl, " Top":dbl}, "Capture 2"=w726:cluster{"Left":dbl, " Top":dbl})
            n528 = Index Array(array=w730, index (row)=0) -> (element=w729:dbl[])  [unwired: 1 in]
            n529 = Index Array(array=w730, index (row)=1) -> (element=w727:dbl[])  [unwired: 1 in]
            n530 = Index Array(array=w727, index=1) -> (element=w749:dbl)
            n531 = Index Array(array=w727, index=0) -> (element=w748:dbl)
            n532 = Index Array(array=w729, index=0) -> (element=w738:dbl)
            n533 = Index Array(array=w729, index=1) -> (element=w739:dbl)
            n534 = expression code="(x*42)+56"(w748) -> (w747:dbl)
            n535 = expression code="(x*42)+469"(w749) -> (w746:dbl)
            n536 = expression code="(x*42)+56"(w738) -> (w740:dbl)
            n537 = expression code="(x*42)+469"(w739) -> (w741:dbl)
            n538 = To Long Integer(number=w746) -> (32bit integer=w745:i32)
            n539 = To Long Integer(number=w747) -> (32bit integer=w744:i32)
            n540 = To Long Integer(number=w741) -> (32bit integer=w742:i32)
            n541 = To Long Integer(number=w740) -> (32bit integer=w743:i32)
            n542 = Bundle(w745, w744) -> (w733:cluster{i32, i32})  [unwired: 1 in]
            n543 = Bundle(w742, w743) -> (w728:cluster{i32, i32})  [unwired: 1 in]
            n544 = property on="P2 Bottom Left Marker" class="Pict"("Position"=w728) -> ()  [unwired: 2 in, 2 out]
            n545 = property on="P2 Bottom Right Marker" class="Pict"("Position"=w733) -> ()  [unwired: 2 in, 2 out]
          }
        }
      }
      event "P2 King", "P2 King 2", "P2 King 3", "P2 King 4", "P2 King 5", "P2 King 6", "P2 King 7", "P2 King 8", "P2 King 9", "P2 King 10", "P2 King 11", "P2 King 12": Mouse Down {
        n546 = event-data() -> ("CtlRef"=w760:refnum<vi>)  [unwired: 1 in, 7 out]
        n547 = local read "P2 Turn Light"() -> (w761:bool)
        n548 = case shown="True" w761 {
          tunnel: w760 -> [_ w765]
          frame False {
            # "It's not player 1's turn yet. Do nothing."
          }
          frame True {
            # "At this point, I use an \nequation to turn the pixel\ncoordinates into the array coordinates\nof the piece that the user clicked."
            # "Left first"
            # "row[0], collumn[1]"
            n549 = property on="Property Node" class="Pict"(reference=w765) -> ("Position"=w766:T1)  [unwired: 1 in, 2 out]
            n550 = global read "Board Layout Global Variable.vi" "Board Layout"() -> (w763:dbl[][])
            n551 = Unbundle By Name(w766) -> ("Left"=w786:i32, "Top"=w784:i32)
            n552 = expression code="(x-469)/42"(w786) -> (w787:i32)
            n553 = expression code="(x-56)/42"(w784) -> (w785:i32)
            n554 = To Long Integer(number=w787) -> (32bit integer=w769:i32)
            n555 = To Long Integer(number=w785) -> (32bit integer=w770:i32)
            n556 = Build Array(w770, w769) -> (w762:i32[])
            n557 = call "MoveLogic.vi"("Array"=w763, "Coordinates"=w762) -> ("Moves"=w764:dbl[][])  [unwired: 2 out]
            n558 = Index Array(array=w764, index (row)=0) -> (element=w771:dbl[])  [unwired: 1 in]
            n559 = Index Array(array=w764, index (row)=1) -> (element=w790:dbl[])  [unwired: 1 in]
            n560 = Index Array(array=w790, index=1) -> (element=w783:dbl)
            n561 = Index Array(array=w790, index=0) -> (element=w782:dbl)
            n562 = Index Array(array=w771, index=0) -> (element=w772:dbl)
            n563 = Index Array(array=w771, index=1) -> (element=w773:dbl)
            n564 = expression code="(x*42)+56"(w782) -> (w781:dbl)
            n565 = expression code="(x*42)+469"(w783) -> (w780:dbl)
            n566 = expression code="(x*42)+56"(w772) -> (w774:dbl)
            n567 = expression code="(x*42)+469"(w773) -> (w775:dbl)
            n568 = To Long Integer(number=w780) -> (32bit integer=w779:i32)
            n569 = To Long Integer(number=w781) -> (32bit integer=w778:i32)
            n570 = To Long Integer(number=w775) -> (32bit integer=w776:i32)
            n571 = To Long Integer(number=w774) -> (32bit integer=w777:i32)
            n572 = Bundle(w779, w778) -> (w768:cluster{i32, i32})  [unwired: 1 in]
            n573 = Bundle(w776, w777) -> (w767:cluster{i32, i32})  [unwired: 1 in]
            n574 = property on="P1 Top Right Marker" class="Pict"("Position"=w768) -> ()  [unwired: 2 in, 2 out]
            n575 = property on="P1 Top Left Marker" class="Pict"("Position"=w767) -> ()  [unwired: 2 in, 2 out]
          }
        }
      }
      event "P1 Top Left Marker": Mouse Down {
        n576 = event-data() -> ()  [unwired: 1 in, 8 out]
        n577 = global read "Board Layout Global Variable.vi" "Board Layout"() -> (w882:dbl[][])
        n578 = property on="P1 Top Left Marker" class="Pict"() -> (error out=w887:errorcluster, "Position"=w889:T1)  [unwired: 2 in, 1 out]
        n579 = call "FixArray.vi"("PreviousState"=w882, "Cluster"=w883, "Array 3"=w884) -> ("NewState"=w881:dbl[][])
        n580 = global write "Board Layout Global Variable.vi" "Board Layout"(w881) -> ()
        n581 = local read "P1 Turn Light"() -> (w877:bool)
        n582 = local read "P1 Turn Light"() -> (w876:bool)
        n583 = local read "P1 Turn Light"() -> (w869:bool)
        n584 = local read "P1 Turn Light"() -> (w865:bool)
        n585 = local read "P1 Turn Light"() -> (w861:bool)
        n586 = local read "P1 Turn Light"() -> (w857:bool)
        n587 = local read "P1 Turn Light"() -> (w856:bool)
        n588 = local read "P1 Turn Light"() -> (w828:bool)
        n589 = local read "P1 Turn Light"() -> (w829:bool)
        n590 = local read "P1 Turn Light"() -> (w836:bool)
        n591 = local read "P1 Turn Light"() -> (w840:bool)
        n592 = local read "P1 Turn Light"() -> (w844:bool)
        n593 = local read "P1 Turn Light"() -> (w848:bool)
        n594 = local read "P1 Turn Light"() -> (w849:bool)
        n595 = local read "P1 Turn Light"() -> (w821:bool)
        n596 = local read "P1 Turn Light"() -> (w820:bool)
        n597 = local read "P1 Turn Light"() -> (w813:bool)
        n598 = local read "P1 Turn Light"() -> (w809:bool)
        n599 = local read "P1 Turn Light"() -> (w805:bool)
        n600 = local read "P1 Turn Light"() -> (w801:bool)
        n601 = local read "P1 Turn Light"() -> (w800:bool)
        n602 = local read "P2 Turn Light"() -> (w879:bool)
        n603 = local read "P2 Turn Light"() -> (w874:bool)
        n604 = local read "P2 Turn Light"() -> (w871:bool)
        n605 = local read "P2 Turn Light"() -> (w867:bool)
        n606 = local read "P2 Turn Light"() -> (w863:bool)
        n607 = local read "P2 Turn Light"() -> (w859:bool)
        n608 = local read "P2 Turn Light"() -> (w854:bool)
        n609 = local read "P2 Turn Light"() -> (w826:bool)
        n610 = local read "P2 Turn Light"() -> (w831:bool)
        n611 = local read "P2 Turn Light"() -> (w834:bool)
        n612 = local read "P2 Turn Light"() -> (w838:bool)
        n613 = local read "P2 Turn Light"() -> (w842:bool)
        n614 = local read "P2 Turn Light"() -> (w846:bool)
        n615 = local read "P2 Turn Light"() -> (w851:bool)
        n616 = local read "P2 Turn Light"() -> (w823:bool)
        n617 = local read "P2 Turn Light"() -> (w818:bool)
        n618 = local read "P2 Turn Light"() -> (w815:bool)
        n619 = local read "P2 Turn Light"() -> (w811:bool)
        n620 = local read "P2 Turn Light"() -> (w807:bool)
        n621 = local read "P2 Turn Light"() -> (w803:bool)
        n622 = local read "P2 Turn Light"() -> (w798:bool)
        n623 = property on="Property Node" class="Pict"(reference=w890, "Position"=w889) -> ()  [unwired: 1 in, 2 out]
        n624 = Not(x=w877) -> (.not. x?=w878:bool)
        n625 = Not(x=w876) -> (.not. x?=w875:bool)
        n626 = Not(x=w869) -> (.not. x?=w870:bool)
        n627 = Not(x=w865) -> (.not. x?=w866:bool)
        n628 = Not(x=w861) -> (.not. x?=w862:bool)
        n629 = Not(x=w857) -> (.not. x?=w858:bool)
        n630 = Not(x=w856) -> (.not. x?=w855:bool)
        n631 = Not(x=w828) -> (.not. x?=w827:bool)
        n632 = Not(x=w829) -> (.not. x?=w830:bool)
        n633 = Not(x=w836) -> (.not. x?=w835:bool)
        n634 = Not(x=w840) -> (.not. x?=w839:bool)
        n635 = Not(x=w844) -> (.not. x?=w843:bool)
        n636 = Not(x=w848) -> (.not. x?=w847:bool)
        n637 = Not(x=w849) -> (.not. x?=w850:bool)
        n638 = Not(x=w821) -> (.not. x?=w822:bool)
        n639 = Not(x=w820) -> (.not. x?=w819:bool)
        n640 = Not(x=w813) -> (.not. x?=w814:bool)
        n641 = Not(x=w809) -> (.not. x?=w810:bool)
        n642 = Not(x=w805) -> (.not. x?=w806:bool)
        n643 = Not(x=w801) -> (.not. x?=w802:bool)
        n644 = Not(x=w800) -> (.not. x?=w799:bool)
        n645 = Not(x=w879) -> (.not. x?=w880:bool)
        n646 = Not(x=w874) -> (.not. x?=w873:bool)
        n647 = Not(x=w871) -> (.not. x?=w872:bool)
        n648 = Not(x=w867) -> (.not. x?=w868:bool)
        n649 = Not(x=w863) -> (.not. x?=w864:bool)
        n650 = Not(x=w859) -> (.not. x?=w860:bool)
        n651 = Not(x=w854) -> (.not. x?=w853:bool)
        n652 = Not(x=w826) -> (.not. x?=w825:bool)
        n653 = Not(x=w831) -> (.not. x?=w832:bool)
        n654 = Not(x=w834) -> (.not. x?=w833:bool)
        n655 = Not(x=w838) -> (.not. x?=w837:bool)
        n656 = Not(x=w842) -> (.not. x?=w841:bool)
        n657 = Not(x=w846) -> (.not. x?=w845:bool)
        n658 = Not(x=w851) -> (.not. x?=w852:bool)
        n659 = Not(x=w823) -> (.not. x?=w824:bool)
        n660 = Not(x=w818) -> (.not. x?=w817:bool)
        n661 = Not(x=w815) -> (.not. x?=w816:bool)
        n662 = Not(x=w811) -> (.not. x?=w812:bool)
        n663 = Not(x=w807) -> (.not. x?=w808:bool)
        n664 = Not(x=w803) -> (.not. x?=w804:bool)
        n665 = Not(x=w798) -> (.not. x?=w797:bool)
        n666 = property on="P1 Bottom Left Marker" class="Pict"("Position"=T1 {"Left"=666, "Top"=666}) -> ()  [unwired: 2 in, 2 out]
        n667 = property on="P1 Bottom Right Marker" class="Pict"("Position"=T1 {"Left"=666, "Top"=666}) -> ()  [unwired: 2 in, 2 out]
        n668 = property on="P1 Top Left Marker" class="Pict"(error in=w887, "Position"=T1 {"Left"=666, "Top"=666}) -> ()  [unwired: 1 in, 2 out]
        n669 = property on="P1 Top Right Marker" class="Pict"("Position"=T1 {"Left"=666, "Top"=666}) -> ()  [unwired: 2 in, 2 out]
        n670 = local write "P2 Turn Light"(w880) -> ()
        n671 = local write "P2 Turn Light"(w873) -> ()
        n672 = local write "P2 Turn Light"(w872) -> ()
        n673 = local write "P2 Turn Light"(w868) -> ()
        n674 = local write "P2 Turn Light"(w864) -> ()
        n675 = local write "P2 Turn Light"(w860) -> ()
        n676 = local write "P2 Turn Light"(w853) -> ()
        n677 = local write "P2 Turn Light"(w825) -> ()
        n678 = local write "P2 Turn Light"(w832) -> ()
        n679 = local write "P2 Turn Light"(w833) -> ()
        n680 = local write "P2 Turn Light"(w837) -> ()
        n681 = local write "P2 Turn Light"(w841) -> ()
        n682 = local write "P2 Turn Light"(w845) -> ()
        n683 = local write "P2 Turn Light"(w852) -> ()
        n684 = local write "P2 Turn Light"(w824) -> ()
        n685 = local write "P2 Turn Light"(w817) -> ()
        n686 = local write "P2 Turn Light"(w816) -> ()
        n687 = local write "P2 Turn Light"(w812) -> ()
        n688 = local write "P2 Turn Light"(w808) -> ()
        n689 = local write "P2 Turn Light"(w804) -> ()
        n690 = local write "P2 Turn Light"(w797) -> ()
        n691 = local write "P1 Turn Light"(w878) -> ()
        n692 = local write "P1 Turn Light"(w875) -> ()
        n693 = local write "P1 Turn Light"(w870) -> ()
        n694 = local write "P1 Turn Light"(w866) -> ()
        n695 = local write "P1 Turn Light"(w862) -> ()
        n696 = local write "P1 Turn Light"(w858) -> ()
        n697 = local write "P1 Turn Light"(w855) -> ()
        n698 = local write "P1 Turn Light"(w827) -> ()
        n699 = local write "P1 Turn Light"(w830) -> ()
        n700 = local write "P1 Turn Light"(w835) -> ()
        n701 = local write "P1 Turn Light"(w839) -> ()
        n702 = local write "P1 Turn Light"(w843) -> ()
        n703 = local write "P1 Turn Light"(w847) -> ()
        n704 = local write "P1 Turn Light"(w850) -> ()
        n705 = local write "P1 Turn Light"(w822) -> ()
        n706 = local write "P1 Turn Light"(w819) -> ()
        n707 = local write "P1 Turn Light"(w814) -> ()
        n708 = local write "P1 Turn Light"(w810) -> ()
        n709 = local write "P1 Turn Light"(w806) -> ()
        n710 = local write "P1 Turn Light"(w802) -> ()
        n711 = local write "P1 Turn Light"(w799) -> ()
        n712 = for {
          tunnel: w796 -> [_] mode=indexing
        }
      }
      event "P2 Top Left Marker": Mouse Down {
        n713 = event-data() -> ()  [unwired: 1 in, 8 out]
        n714 = property on="P2 Top Left Marker" class="Pict"() -> (error out=w898:errorcluster, "Position"=w899:T1)  [unwired: 2 in, 1 out]
        n715 = local read "P1 Turn Light"() -> (w894:bool)
        n716 = property on="Property Node" class="Pict"(reference=w901, "Position"=w899) -> ()  [unwired: 1 in, 2 out]
        n717 = local read "P2 Turn Light"() -> (w892:bool)
        n718 = Not(x=w894) -> (.not. x?=w893:bool)
        n719 = Not(x=w892) -> (.not. x?=w891:bool)
        n720 = local write "P2 Turn Light"(w891) -> ()
        n721 = property on="P2 Bottom Right Marker" class="Pict"("Position"=T1 {"Left"=666, "Top"=666}) -> ()  [unwired: 2 in, 2 out]
        n722 = property on="P2 Top Left Marker" class="Pict"(error in=w898, "Position"=T1 {"Left"=666, "Top"=666}) -> ()  [unwired: 1 in, 2 out]
        n723 = property on="P2 Top Right Marker" class="Pict"("Position"=T1 {"Left"=666, "Top"=666}) -> ()  [unwired: 2 in, 2 out]
        n724 = local write "P1 Turn Light"(w893) -> ()
        n725 = property on="P2 Bottom Left Marker" class="Pict"("Position"=T1 {"Left"=666, "Top"=666}) -> ()  [unwired: 2 in, 2 out]
      }
      event "P2 Top Right Marker": Mouse Down {
        n726 = event-data() -> ()  [unwired: 1 in, 8 out]
        n727 = property on="P2 Top Right Marker" class="Pict"() -> (error out=w906:errorcluster, "Position"=w907:T1)  [unwired: 2 in, 1 out]
        n728 = local read "P1 Turn Light"() -> (w905:bool)
        n729 = local read "P2 Turn Light"() -> (w903:bool)
        n730 = property on="Property Node" class="Pict"(reference=w912, "Position"=w907) -> ()  [unwired: 1 in, 2 out]
        n731 = Not(x=w905) -> (.not. x?=w904:bool)
        n732 = Not(x=w903) -> (.not. x?=w902:bool)
        n733 = local write "P2 Turn Light"(w902) -> ()
        n734 = local write "P1 Turn Light"(w904) -> ()
        n735 = property on="P2 Bottom Right Marker" class="Pict"("Position"=T1 {"Left"=666, "Top"=666}) -> ()  [unwired: 2 in, 2 out]
        n736 = property on="P2 Top Left Marker" class="Pict"("Position"=T1 {"Left"=666, "Top"=666}) -> ()  [unwired: 2 in, 2 out]
        n737 = property on="P2 Top Right Marker" class="Pict"(error in=w906, "Position"=T1 {"Left"=666, "Top"=666}) -> ()  [unwired: 1 in, 2 out]
        n738 = property on="P2 Bottom Left Marker" class="Pict"("Position"=T1 {"Left"=666, "Top"=666}) -> ()  [unwired: 2 in, 2 out]
      }
      event "P2 Bottom Left Marker": Mouse Down {
        n739 = event-data() -> ()  [unwired: 1 in, 8 out]
        n740 = property on="P2 Bottom Left Marker" class="Pict"() -> (error out=w917:errorcluster, "Position"=w918:T1)  [unwired: 2 in, 1 out]
        n741 = local read "P1 Turn Light"() -> (w916:bool)
        n742 = local read "P2 Turn Light"() -> (w914:bool)
        n743 = property on="Property Node" class="Pict"(reference=w923, "Position"=w918) -> ()  [unwired: 1 in, 2 out]
        n744 = Not(x=w916) -> (.not. x?=w915:bool)
        n745 = Not(x=w914) -> (.not. x?=w913:bool)
        n746 = local write "P2 Turn Light"(w913) -> ()
        n747 = local write "P1 Turn Light"(w915) -> ()
        n748 = property on="P2 Bottom Right Marker" class="Pict"("Position"=T1 {"Left"=666, "Top"=666}) -> ()  [unwired: 2 in, 2 out]
        n749 = property on="P2 Top Left Marker" class="Pict"("Position"=T1 {"Left"=666, "Top"=666}) -> ()  [unwired: 2 in, 2 out]
        n750 = property on="P2 Top Right Marker" class="Pict"("Position"=T1 {"Left"=666, "Top"=666}) -> ()  [unwired: 2 in, 2 out]
        n751 = property on="P2 Bottom Left Marker" class="Pict"(error in=w917, "Position"=T1 {"Left"=666, "Top"=666}) -> ()  [unwired: 1 in, 2 out]
      }
      event "P2 Bottom Right Marker": Mouse Down {
        n752 = event-data() -> ()  [unwired: 1 in, 8 out]
        n753 = property on="P2 Bottom Right Marker" class="Pict"() -> (error out=w928:errorcluster, "Position"=w929:T1)  [unwired: 2 in, 1 out]
        n754 = local read "P1 Turn Light"() -> (w927:bool)
        n755 = property on="Property Node" class="Pict"(reference=w934, "Position"=w929) -> ()  [unwired: 1 in, 2 out]
        n756 = local read "P2 Turn Light"() -> (w925:bool)
        n757 = Not(x=w927) -> (.not. x?=w926:bool)
        n758 = Not(x=w925) -> (.not. x?=w924:bool)
        n759 = local write "P2 Turn Light"(w924) -> ()
        n760 = property on="P2 Bottom Right Marker" class="Pict"(error in=w928, "Position"=T1 {"Left"=666, "Top"=666}) -> ()  [unwired: 1 in, 2 out]
        n761 = property on="P2 Top Left Marker" class="Pict"("Position"=T1 {"Left"=666, "Top"=666}) -> ()  [unwired: 2 in, 2 out]
        n762 = property on="P2 Top Right Marker" class="Pict"("Position"=T1 {"Left"=666, "Top"=666}) -> ()  [unwired: 2 in, 2 out]
        n763 = property on="P2 Bottom Left Marker" class="Pict"("Position"=T1 {"Left"=666, "Top"=666}) -> ()  [unwired: 2 in, 2 out]
        n764 = local write "P1 Turn Light"(w926) -> ()
      }
      event "P1 Top Right Marker": Mouse Down {
        n765 = event-data() -> ()  [unwired: 1 in, 8 out]
        n766 = property on="P1 Top Right Marker" class="Pict"() -> ("Position"=w944:T1)  [unwired: 2 in, 2 out]
        n767 = global read "Board Layout Global Variable.vi" "Board Layout"() -> (w938:dbl[][])
        n768 = call "FixArray.vi"("PreviousState"=w938, "Cluster"=w936, "Array 3"=w935) -> ("NewState"=w937:dbl[][])
        n769 = global write "Board Layout Global Variable.vi" "Board Layout"(w937) -> ()
        n770 = property on="Property Node" class="Pict"(reference=w949, "Position"=w944) -> (error out=w943:errorcluster)  [unwired: 1 in, 1 out]
        n771 = property on="P1 Bottom Left Marker" class="Pict"("Position"=T1 {"Left"=666, "Top"=666}) -> ()  [unwired: 2 in, 2 out]
        n772 = property on="P1 Bottom Right Marker" class="Pict"("Position"=T1 {"Left"=666, "Top"=666}) -> ()  [unwired: 2 in, 2 out]
        n773 = property on="P1 Top Left Marker" class="Pict"("Position"=T1 {"Left"=666, "Top"=666}) -> ()  [unwired: 2 in, 2 out]
        n774 = property on="P1 Top Right Marker" class="Pict"(error in=w943, "Position"=T1 {"Left"=666, "Top"=666}) -> ()  [unwired: 1 in, 2 out]
        n775 = local read "P1 Turn Light"() -> (w942:bool)
        n776 = local read "P2 Turn Light"() -> (w940:bool)
        n777 = Not(x=w942) -> (.not. x?=w941:bool)
        n778 = Not(x=w940) -> (.not. x?=w939:bool)
        n779 = local write "P2 Turn Light"(w939) -> ()
        n780 = local write "P1 Turn Light"(w941) -> ()
      }
      event "P1 Bottom Left Marker": Mouse Down {
        n781 = event-data() -> ()  [unwired: 1 in, 8 out]
        n782 = property on="P1 Bottom Left Marker" class="Pict"() -> ("Position"=w979:T1)  [unwired: 2 in, 2 out]
        n783 = local read "P1 Turn Light"() -> (w974:bool)
        n784 = local read "P1 Turn Light"() -> (w973:bool)
        n785 = local read "P1 Turn Light"() -> (w966:bool)
        n786 = local read "P1 Turn Light"() -> (w962:bool)
        n787 = local read "P1 Turn Light"() -> (w958:bool)
        n788 = local read "P1 Turn Light"() -> (w954:bool)
        n789 = local read "P1 Turn Light"() -> (w953:bool)
        n790 = local read "P2 Turn Light"() -> (w976:bool)
        n791 = local read "P2 Turn Light"() -> (w971:bool)
        n792 = local read "P2 Turn Light"() -> (w968:bool)
        n793 = local read "P2 Turn Light"() -> (w964:bool)
        n794 = local read "P2 Turn Light"() -> (w960:bool)
        n795 = local read "P2 Turn Light"() -> (w956:bool)
        n796 = local read "P2 Turn Light"() -> (w951:bool)
        n797 = property on="Property Node" class="Pict"(reference=w984, "Position"=w979) -> (error out=w978:errorcluster)  [unwired: 1 in, 1 out]
        n798 = Not(x=w974) -> (.not. x?=w975:bool)
        n799 = Not(x=w973) -> (.not. x?=w972:bool)
        n800 = Not(x=w966) -> (.not. x?=w967:bool)
        n801 = Not(x=w962) -> (.not. x?=w963:bool)
        n802 = Not(x=w958) -> (.not. x?=w959:bool)
        n803 = Not(x=w954) -> (.not. x?=w955:bool)
        n804 = Not(x=w953) -> (.not. x?=w952:bool)
        n805 = Not(x=w976) -> (.not. x?=w977:bool)
        n806 = Not(x=w971) -> (.not. x?=w970:bool)
        n807 = Not(x=w968) -> (.not. x?=w969:bool)
        n808 = Not(x=w964) -> (.not. x?=w965:bool)
        n809 = Not(x=w960) -> (.not. x?=w961:bool)
        n810 = Not(x=w956) -> (.not. x?=w957:bool)
        n811 = Not(x=w951) -> (.not. x?=w950:bool)
        n812 = local write "P2 Turn Light"(w977) -> ()
        n813 = local write "P2 Turn Light"(w970) -> ()
        n814 = local write "P2 Turn Light"(w969) -> ()
        n815 = local write "P2 Turn Light"(w965) -> ()
        n816 = local write "P2 Turn Light"(w961) -> ()
        n817 = local write "P2 Turn Light"(w957) -> ()
        n818 = local write "P2 Turn Light"(w950) -> ()
        n819 = local write "P1 Turn Light"(w975) -> ()
        n820 = local write "P1 Turn Light"(w972) -> ()
        n821 = local write "P1 Turn Light"(w967) -> ()
        n822 = local write "P1 Turn Light"(w963) -> ()
        n823 = local write "P1 Turn Light"(w959) -> ()
        n824 = local write "P1 Turn Light"(w955) -> ()
        n825 = local write "P1 Turn Light"(w952) -> ()
        n826 = property on="P1 Bottom Left Marker" class="Pict"(error in=w978, "Position"=T1 {"Left"=666, "Top"=666}) -> ()  [unwired: 1 in, 2 out]
        n827 = property on="P1 Bottom Right Marker" class="Pict"("Position"=T1 {"Left"=666, "Top"=666}) -> ()  [unwired: 2 in, 2 out]
        n828 = property on="P1 Top Left Marker" class="Pict"("Position"=T1 {"Left"=666, "Top"=666}) -> ()  [unwired: 2 in, 2 out]
        n829 = property on="P1 Top Right Marker" class="Pict"("Position"=T1 {"Left"=666, "Top"=666}) -> ()  [unwired: 2 in, 2 out]
      }
      event "P1 Bottom Right Marker": Mouse Down {
        n830 = event-data() -> ()  [unwired: 1 in, 8 out]
        n831 = property on="P1 Bottom Right Marker" class="Pict"() -> ("Position"=w1070:T1)  [unwired: 2 in, 2 out]
        n832 = local read "P1 Turn Light"() -> (w1065:bool)
        n833 = local read "P1 Turn Light"() -> (w1064:bool)
        n834 = local read "P1 Turn Light"() -> (w1057:bool)
        n835 = local read "P1 Turn Light"() -> (w1053:bool)
        n836 = local read "P1 Turn Light"() -> (w1049:bool)
        n837 = local read "P1 Turn Light"() -> (w1045:bool)
        n838 = local read "P1 Turn Light"() -> (w1044:bool)
        n839 = local read "P1 Turn Light"() -> (w1016:bool)
        n840 = local read "P1 Turn Light"() -> (w1017:bool)
        n841 = local read "P1 Turn Light"() -> (w1024:bool)
        n842 = local read "P1 Turn Light"() -> (w1028:bool)
        n843 = local read "P1 Turn Light"() -> (w1032:bool)
        n844 = local read "P1 Turn Light"() -> (w1036:bool)
        n845 = local read "P1 Turn Light"() -> (w1037:bool)
        n846 = local read "P1 Turn Light"() -> (w1009:bool)
        n847 = local read "P1 Turn Light"() -> (w1008:bool)
        n848 = local read "P1 Turn Light"() -> (w1001:bool)
        n849 = local read "P1 Turn Light"() -> (w997:bool)
        n850 = local read "P1 Turn Light"() -> (w993:bool)
        n851 = local read "P1 Turn Light"() -> (w989:bool)
        n852 = local read "P1 Turn Light"() -> (w988:bool)
        n853 = local read "P2 Turn Light"() -> (w1067:bool)
        n854 = local read "P2 Turn Light"() -> (w1062:bool)
        n855 = local read "P2 Turn Light"() -> (w1059:bool)
        n856 = local read "P2 Turn Light"() -> (w1055:bool)
        n857 = local read "P2 Turn Light"() -> (w1051:bool)
        n858 = local read "P2 Turn Light"() -> (w1047:bool)
        n859 = local read "P2 Turn Light"() -> (w1042:bool)
        n860 = local read "P2 Turn Light"() -> (w1014:bool)
        n861 = local read "P2 Turn Light"() -> (w1019:bool)
        n862 = local read "P2 Turn Light"() -> (w1022:bool)
        n863 = local read "P2 Turn Light"() -> (w1026:bool)
        n864 = local read "P2 Turn Light"() -> (w1030:bool)
        n865 = local read "P2 Turn Light"() -> (w1034:bool)
        n866 = local read "P2 Turn Light"() -> (w1039:bool)
        n867 = local read "P2 Turn Light"() -> (w1011:bool)
        n868 = local read "P2 Turn Light"() -> (w1006:bool)
        n869 = local read "P2 Turn Light"() -> (w1003:bool)
        n870 = local read "P2 Turn Light"() -> (w999:bool)
        n871 = local read "P2 Turn Light"() -> (w995:bool)
        n872 = local read "P2 Turn Light"() -> (w991:bool)
        n873 = local read "P2 Turn Light"() -> (w986:bool)
        n874 = property on="Property Node" class="Pict"(reference=w1075, "Position"=w1070) -> (error out=w1069:errorcluster)  [unwired: 1 in, 1 out]
        n875 = Not(x=w1065) -> (.not. x?=w1066:bool)
        n876 = Not(x=w1064) -> (.not. x?=w1063:bool)
        n877 = Not(x=w1057) -> (.not. x?=w1058:bool)
        n878 = Not(x=w1053) -> (.not. x?=w1054:bool)
        n879 = Not(x=w1049) -> (.not. x?=w1050:bool)
        n880 = Not(x=w1045) -> (.not. x?=w1046:bool)
        n881 = Not(x=w1044) -> (.not. x?=w1043:bool)
        n882 = Not(x=w1016) -> (.not. x?=w1015:bool)
        n883 = Not(x=w1017) -> (.not. x?=w1018:bool)
        n884 = Not(x=w1024) -> (.not. x?=w1023:bool)
        n885 = Not(x=w1028) -> (.not. x?=w1027:bool)
        n886 = Not(x=w1032) -> (.not. x?=w1031:bool)
        n887 = Not(x=w1036) -> (.not. x?=w1035:bool)
        n888 = Not(x=w1037) -> (.not. x?=w1038:bool)
        n889 = Not(x=w1009) -> (.not. x?=w1010:bool)
        n890 = Not(x=w1008) -> (.not. x?=w1007:bool)
        n891 = Not(x=w1001) -> (.not. x?=w1002:bool)
        n892 = Not(x=w997) -> (.not. x?=w998:bool)
        n893 = Not(x=w993) -> (.not. x?=w994:bool)
        n894 = Not(x=w989) -> (.not. x?=w990:bool)
        n895 = Not(x=w988) -> (.not. x?=w987:bool)
        n896 = Not(x=w1067) -> (.not. x?=w1068:bool)
        n897 = Not(x=w1062) -> (.not. x?=w1061:bool)
        n898 = Not(x=w1059) -> (.not. x?=w1060:bool)
        n899 = Not(x=w1055) -> (.not. x?=w1056:bool)
        n900 = Not(x=w1051) -> (.not. x?=w1052:bool)
        n901 = Not(x=w1047) -> (.not. x?=w1048:bool)
        n902 = Not(x=w1042) -> (.not. x?=w1041:bool)
        n903 = Not(x=w1014) -> (.not. x?=w1013:bool)
        n904 = Not(x=w1019) -> (.not. x?=w1020:bool)
        n905 = Not(x=w1022) -> (.not. x?=w1021:bool)
        n906 = Not(x=w1026) -> (.not. x?=w1025:bool)
        n907 = Not(x=w1030) -> (.not. x?=w1029:bool)
        n908 = Not(x=w1034) -> (.not. x?=w1033:bool)
        n909 = Not(x=w1039) -> (.not. x?=w1040:bool)
        n910 = Not(x=w1011) -> (.not. x?=w1012:bool)
        n911 = Not(x=w1006) -> (.not. x?=w1005:bool)
        n912 = Not(x=w1003) -> (.not. x?=w1004:bool)
        n913 = Not(x=w999) -> (.not. x?=w1000:bool)
        n914 = Not(x=w995) -> (.not. x?=w996:bool)
        n915 = Not(x=w991) -> (.not. x?=w992:bool)
        n916 = Not(x=w986) -> (.not. x?=w985:bool)
        n917 = local write "P2 Turn Light"(w1068) -> ()
        n918 = local write "P2 Turn Light"(w1061) -> ()
        n919 = local write "P2 Turn Light"(w1060) -> ()
        n920 = local write "P2 Turn Light"(w1056) -> ()
        n921 = local write "P2 Turn Light"(w1052) -> ()
        n922 = local write "P2 Turn Light"(w1048) -> ()
        n923 = local write "P2 Turn Light"(w1041) -> ()
        n924 = local write "P2 Turn Light"(w1013) -> ()
        n925 = local write "P2 Turn Light"(w1020) -> ()
        n926 = local write "P2 Turn Light"(w1021) -> ()
        n927 = local write "P2 Turn Light"(w1025) -> ()
        n928 = local write "P2 Turn Light"(w1029) -> ()
        n929 = local write "P2 Turn Light"(w1033) -> ()
        n930 = local write "P2 Turn Light"(w1040) -> ()
        n931 = local write "P2 Turn Light"(w1012) -> ()
        n932 = local write "P2 Turn Light"(w1005) -> ()
        n933 = local write "P2 Turn Light"(w1004) -> ()
        n934 = local write "P2 Turn Light"(w1000) -> ()
        n935 = local write "P2 Turn Light"(w996) -> ()
        n936 = local write "P2 Turn Light"(w992) -> ()
        n937 = local write "P2 Turn Light"(w985) -> ()
        n938 = local write "P1 Turn Light"(w1066) -> ()
        n939 = local write "P1 Turn Light"(w1063) -> ()
        n940 = local write "P1 Turn Light"(w1058) -> ()
        n941 = local write "P1 Turn Light"(w1054) -> ()
        n942 = local write "P1 Turn Light"(w1050) -> ()
        n943 = local write "P1 Turn Light"(w1046) -> ()
        n944 = local write "P1 Turn Light"(w1043) -> ()
        n945 = local write "P1 Turn Light"(w1015) -> ()
        n946 = local write "P1 Turn Light"(w1018) -> ()
        n947 = local write "P1 Turn Light"(w1023) -> ()
        n948 = local write "P1 Turn Light"(w1027) -> ()
        n949 = local write "P1 Turn Light"(w1031) -> ()
        n950 = local write "P1 Turn Light"(w1035) -> ()
        n951 = local write "P1 Turn Light"(w1038) -> ()
        n952 = local write "P1 Turn Light"(w1010) -> ()
        n953 = local write "P1 Turn Light"(w1007) -> ()
        n954 = local write "P1 Turn Light"(w1002) -> ()
        n955 = local write "P1 Turn Light"(w998) -> ()
        n956 = local write "P1 Turn Light"(w994) -> ()
        n957 = local write "P1 Turn Light"(w990) -> ()
        n958 = local write "P1 Turn Light"(w987) -> ()
        n959 = property on="P1 Top Left Marker" class="Pict"("Position"=T1 {"Left"=666, "Top"=666}) -> ()  [unwired: 2 in, 2 out]
        n960 = property on="P1 Top Right Marker" class="Pict"("Position"=T1 {"Left"=666, "Top"=666}) -> ()  [unwired: 2 in, 2 out]
        n961 = property on="P1 Bottom Right Marker" class="Pict"(error in=w1069, "Position"=T1 {"Left"=666, "Top"=666}) -> ()  [unwired: 1 in, 2 out]
        n962 = property on="P1 Bottom Left Marker" class="Pict"("Position"=T1 {"Left"=666, "Top"=666}) -> ()  [unwired: 2 in, 2 out]
      }
    }
  }
  n963 = stacked-sequence {
    frame #0 {
      n964 = call "Checkers P1 Turn Drawer.vi"() -> ("new picture"=→"P1 Top Right Marker":picture)  [unwired: 11 in]
      n965 = property on="P1 Top Right Marker" class="Pict"("Position"=T1 {"Left"=666, "Top"=666}) -> ()  [unwired: 2 in, 2 out]
    }
    frame #1 {
      n966 = call "Checkers P1 Turn Drawer.vi"() -> ("new picture"=→"P1 Top Left Marker":picture)  [unwired: 11 in]
      n967 = property on="P1 Top Left Marker" class="Pict"("Position"=T1 {"Left"=666, "Top"=666}) -> ()  [unwired: 2 in, 2 out]
    }
    frame #2 {
      n968 = call "Checkers P1 Turn Drawer.vi"() -> ("new picture"=→"P1 Bottom Left Marker":picture)  [unwired: 11 in]
      n969 = property on="P1 Bottom Left Marker" class="Pict"("Position"=T1 {"Left"=666, "Top"=666}) -> ()  [unwired: 2 in, 2 out]
    }
    frame #3 {
      n970 = call "Checkers P1 Turn Drawer.vi"() -> ("new picture"=→"P1 Bottom Right Marker":picture)  [unwired: 11 in]
      n971 = property on="P1 Bottom Right Marker" class="Pict"("Position"=T1 {"Left"=666, "Top"=666}) -> ()  [unwired: 2 in, 2 out]
    }
    frame #4 {
      n972 = call "Checkers P2 Turn Drawer.vi"() -> ("new picture"=→"P2 Top Left Marker":picture)  [unwired: 11 in]
      n973 = property on="P2 Top Left Marker" class="Pict"("Position"=T1 {"Left"=666, "Top"=666}) -> ()  [unwired: 2 in, 2 out]
    }
    frame #5 {
      n974 = call "Checkers P2 Turn Drawer.vi"() -> ("new picture"=→"P2 Top Right Marker":picture)  [unwired: 11 in]
      n975 = property on="P2 Top Right Marker" class="Pict"("Position"=T1 {"Left"=666, "Top"=666}) -> ()  [unwired: 2 in, 2 out]
    }
    frame #6 {
      n976 = call "Checkers P2 Turn Drawer.vi"() -> ("new picture"=→"P2 Bottom Left Marker":picture)  [unwired: 11 in]
      n977 = property on="P2 Bottom Left Marker" class="Pict"("Position"=T1 {"Left"=666, "Top"=666}) -> ()  [unwired: 2 in, 2 out]
    }
    frame #7 {
      n978 = call "Checkers P2 Turn Drawer.vi"() -> ("new picture"=→"P2 Bottom Right Marker":picture)  [unwired: 11 in]
      n979 = property on="P2 Bottom Right Marker" class="Pict"("Position"=T1 {"Left"=666, "Top"=666}) -> ()  [unwired: 2 in, 2 out]
    }
  }
  "Player 1 Label" <- "Player 1" ("String 3")
  "Player 2 Label" <- "Player 2" ("String 4")
